vi "PJ_Edit_Freq.vi"() -> ()   [LabVIEW 2025]
uses:
  <vilib>/express/express analysis/Spectral/Block/exnSpectralBlock spectral measurements PSD poly.vi
  <vilib>/express/express analysis/Spectral/Block/exnSpectralBlock spectral measurements PSD DDT.vi
  <vilib>/express/express analysis/Spectral/XNode/ExpressSpectralMeasurementsBlockNode.xnode
panel:
  in  "start":bool
  in  "Boolean":bool
  in  "Fre":dbl
  in  "Am":dbl
  out "Clear4":bool
  out "Clear 3":bool
  out "Clear2":bool
  out "check":bool
  out "Clear1":bool
  out "com":bool
  out "call":bool
  out "ele":bool
  in  "Baseline":bool
  out "555":bool
  out "6 HZ 2":bool
  out "7 HZ":bool
  in  "Upper Cut-Off":dbl=40.0
  out "PSD":dynamicdata(graph)
  out "PSD MAX":dbl
  out "Index ที่มากที่สุด":i32
  out "max value":dbl
  out "B 22+1":dbl
  out "N 22+1":dbl
  in  "Aj 22+1":dbl
  out "B 22+1":dbl
  out "PSD 22+1":dbl
  out "B 22":dbl
  out "N 22":dbl
  in  "Aj 22":dbl
  out "B 22":dbl
  out "PSD 22":dbl
  out "B 22-1":dbl
  out "N 22-1":dbl
  in  "Aj 22-1":dbl
  out "B 22-1":dbl
  out "PSD 22-1":dbl
  out "9 Hz":dbl[](array[numeric])
  out "Max Index 9":i32
  out "PSD max 9":dbl
  out "PSD 11-1":dbl
  out "B 11-1":dbl
  in  "Aj 11-1":dbl
  out "N 11-1":dbl
  out "B 11-1":dbl
  out "PSD 11":dbl
  out "B 11":dbl
  in  "Aj 11":dbl
  out "N 11":dbl
  out "B 11":dbl
  out "PSD 11+1":dbl
  out "B 11+1":dbl
  in  "Aj 11+1":dbl
  out "N 11+1":dbl
  out "B 11+1":dbl
  out "8 Hz":dbl[](array[numeric])
  out "Max Index 8":i32
  out "PSD max 8":dbl
  out "B 16+1":dbl
  out "N 16+1":dbl
  in  "Aj  16+1":dbl
  out "B 16+1":dbl
  out "PSD  16+1":dbl
  out "B 16":dbl
  out "N  16":dbl
  in  "Aj  16":dbl
  out "B 16":dbl
  out "PSD  16":dbl
  out "B 16-1":dbl
  out "N  16-1":dbl
  in  "Aj   16-1":dbl
  out "B   16-1":dbl
  out "PSD 16-1":dbl
  out "B 8+1":dbl
  out "N 8+1":dbl
  in  "Aj  8+1":dbl
  out "B  8+1":dbl
  out "PSD 8+1":dbl
  out "B 8":dbl
  out "N  8":dbl
  in  "Aj  8":dbl
  out "B  8":dbl
  out "PSD 8":dbl
  out "B 8-1":dbl
  out "N  8-1":dbl
  in  "Aj  8-1":dbl
  out "B  8-1":dbl
  out "PSD 8-1":dbl
  out "PSD 14+1":dbl
  out "B 14+1":dbl
  in  "Aj 14+1":dbl
  out "N 14+1":dbl
  out "B 14+1":dbl
  out "PSD 14":dbl
  out "B 14":dbl
  in  "Aj 14":dbl
  out "N 14":dbl
  out "B 14":dbl
  out "PSD 14-1":dbl
  out "B 14-1":dbl
  in  "Aj 14-1":dbl
  out "N 14-1":dbl
  out "B 14-1":dbl
  out "PSD7+1":dbl
  out "B7+1":dbl
  in  "Aj7+1":dbl
  out "N7+1":dbl
  out "B7+1":dbl
  out "PSD 7":dbl
  out "B 7":dbl
  in  "Aj 7":dbl
  out "N7":dbl
  out "B7":dbl
  out "7 Hz":dbl[](array[numeric])
  out "Max Index 7":i32
  out "PSD max 7":dbl
  out "PSD 7-1":dbl
  out "B 7-1":dbl
  in  "Aj 7-1":dbl
  out "N7-1":dbl
  out "B7-1":dbl
  out "B12-1":dbl
  out "N12-1":dbl
  in  "Aj 12-1":dbl
  out "B 12-1":dbl
  out "PSD 12-1":dbl
  out "B12":dbl
  out "N12":dbl
  in  "Aj 12":dbl
  out "B12":dbl
  out "PSD 12":dbl
  out "B12+1":dbl
  out "N12+1":dbl
  in  "Aj 12+1":dbl
  out "B 12+1":dbl
  out "PSD 12+1":dbl
  out "B6+1":dbl
  out "N6+1":dbl
  in  "Aj 6+1":dbl
  out "B 6+1":dbl
  out "PSD 6+1":dbl
  out "B6":dbl
  out "N6":dbl
  in  "Aj 6":dbl
  out "B6":dbl
  out "PSD 6":dbl
  out "PSD 6-1":dbl
  out "6 Hz":dbl[](array[numeric])
  out "Max Index 6":i32
  out "PSD max 6":dbl
  out "B 6-1":dbl
  in  "Aj 6-1":dbl
  out "N6-1":dbl
  out "B6-1":dbl
  out "appended array":dbl[][](array[numeric])
  out "Filtered Signal":dynamicdata(graph)
  in  "Lower Cut-Off":dbl=1.0
  out "data":dynamicdata(graph) caption="Raw Data"
  in  "number of samples":i32=1000
  in  "rate":dbl=200.0 min=200.0 max=200.0
  out "?":bool
  out "?":bool
  out "?":bool
  out "?":bool
  out "?":bool
  out "?":bool
  out "?":bool
  out "?":bool
  out "?":bool
  out "?":bool
  out "?":bool=TRUE
  out "?":bool=TRUE
  out "?":bool=TRUE
  out "?":bool=TRUE
  out "?":bool=TRUE
  out "?":bool=TRUE
  out "?":bool=TRUE
  out "?":bool=TRUE
  out "?":bool=TRUE
  out "?":bool=TRUE
  out "?":bool
  out "?":bool
  out "?":bool
  out "?":bool
  out "?":bool
  out "?":bool
  out "?":bool
  out "?":bool
  out "?":bool
  out "?":bool
  out "?":bool=TRUE
  out "?":bool=TRUE
  out "?":bool=TRUE
  out "?":bool=TRUE
  out "?":bool=TRUE
  out "?":bool=TRUE
  out "?":bool=TRUE
  out "?":bool=TRUE
  out "?":bool=TRUE
  out "?":bool=TRUE
  out "?":bool
  out "?":bool
  out "?":bool
  out "?":bool
  out "?":bool
  out "?":bool
  out "?":bool
  out "?":bool
  out "?":bool
  out "?":bool
  out "?":bool=TRUE
  out "?":bool=TRUE
  out "?":bool=TRUE
  out "?":bool=TRUE
  out "?":bool=TRUE
  out "?":bool=TRUE
  out "?":bool=TRUE
  out "?":bool=TRUE
  out "?":bool=TRUE
  out "?":bool=TRUE
  out "?":bool
  out "?":bool
  out "?":bool
  out "?":bool
  out "?":bool
  out "?":bool
  out "?":bool
  out "?":bool
  out "?":bool
  out "?":bool
  out "?":bool=TRUE
  out "?":bool=TRUE
  out "?":bool=TRUE
  out "?":bool=TRUE
  out "?":bool=TRUE
  out "?":bool=TRUE
  out "?":bool=TRUE
  out "?":bool=TRUE
  out "?":bool=TRUE
  out "?":bool=TRUE
  out "9 HZ":bool
  out "8 HZ":bool
  in  "Tab Control":enum32{"TAB 1", "TAB 2", "TAB 3", "TAB 4"}(tab)
  out "Emotion 7":bool
  out "Emotion 6":bool
  out "Emotion 5":bool
  out "Emotion 4":bool
  out "ele":bool
  out "Emer":bool
  out "call":bool
  out "commu":bool
  out "Activity":bool
  out "8-2":bool
  out "commu_back":bool
  out "commu_2":bool
  out "commu_1":bool
  out "Emotion":bool
  out "ACC":bool
  out "back_page2":bool
  in  "send":bool
  out "call_back":bool
  out "call_3":bool
  out "call_back":bool
  out "call_2":bool
  out "call_1":bool
  out "1 3":bool
  out "1 2":bool
  out "1":bool
  out "String 2":string
  in  "SOS CALLING":bool
  in  "Search Button 2":bool
  out "ele_back":bool
  out "ele_3":bool
  out "ele_2":bool
  out "ele_1":bool
  out "ele_2":bool
  out "ele_3":bool
  out "ele_1":bool
  out "BACK_Page4":bool
  # "MENU"
  # "COMMUNICATION"
  # "SOS CALLING"
  # "Tel."
  # "ELECTRICAL DEVICES"
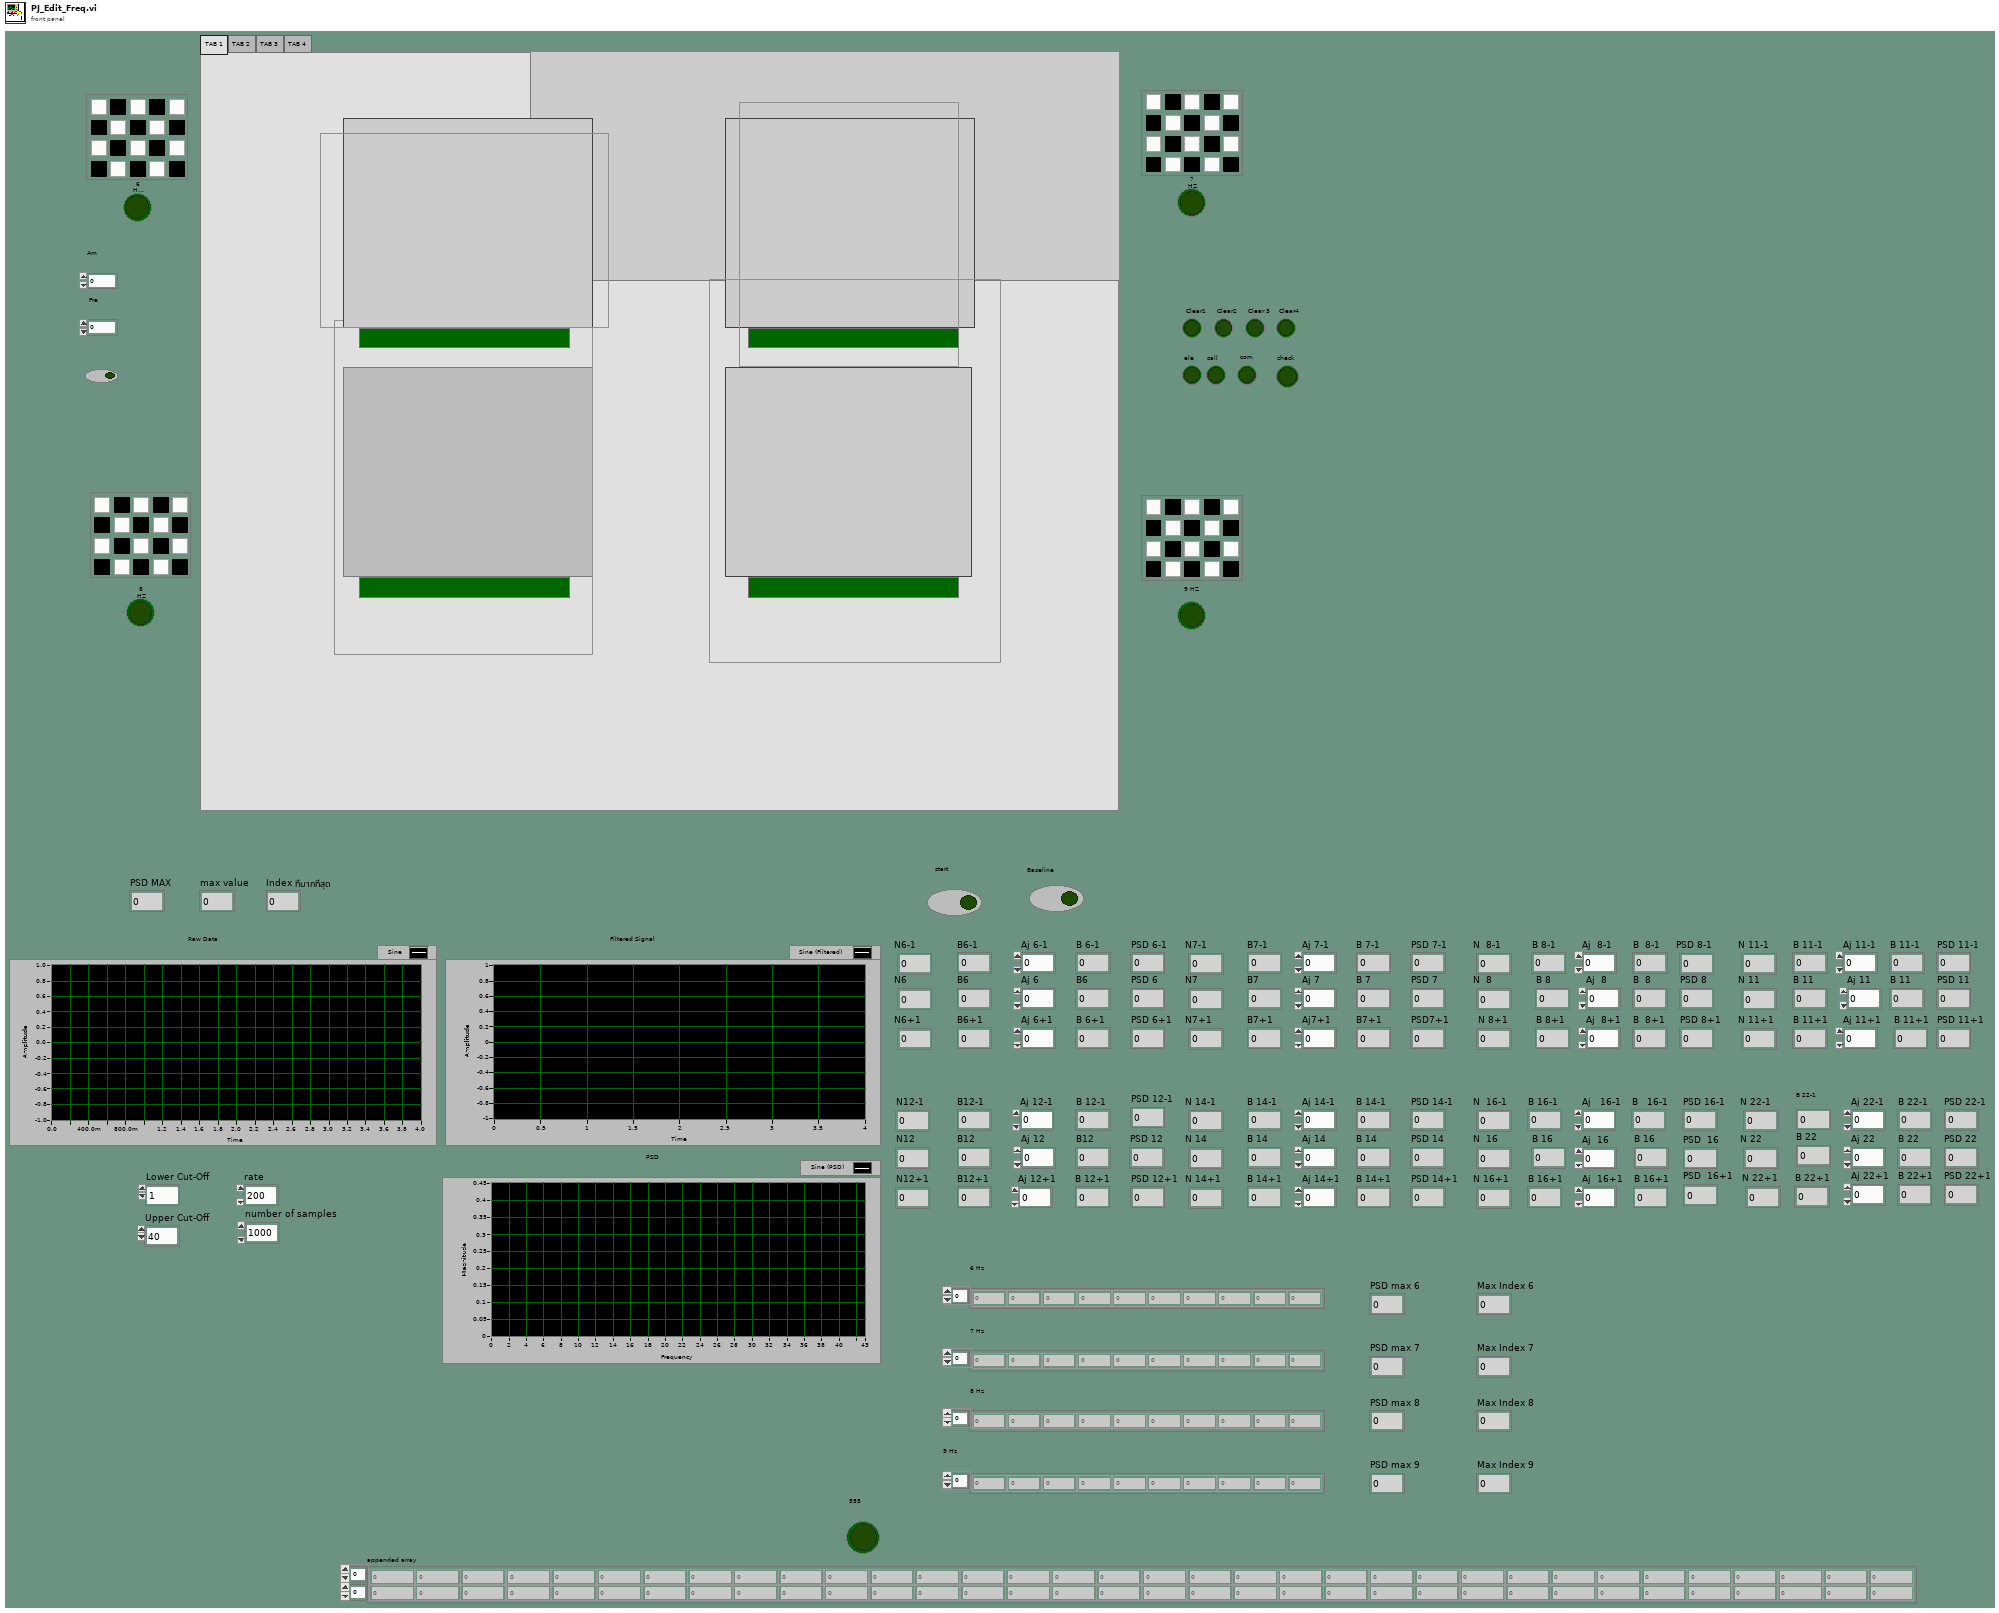
[diagram p1: front panel]
types:
  T1 = cluster{"averaging mode":u16, "weighting mode":u16, "number of averages":u32}
  T2 = cluster{"dB On (F)":bool, "unwrap phase (F)":bool, "convert to degree (F)":bool}
  T3 = enum32{"TAB 1", "TAB 2", "TAB 3", "TAB 4", "TAB 5", "TAB 6", "TAB 7"}
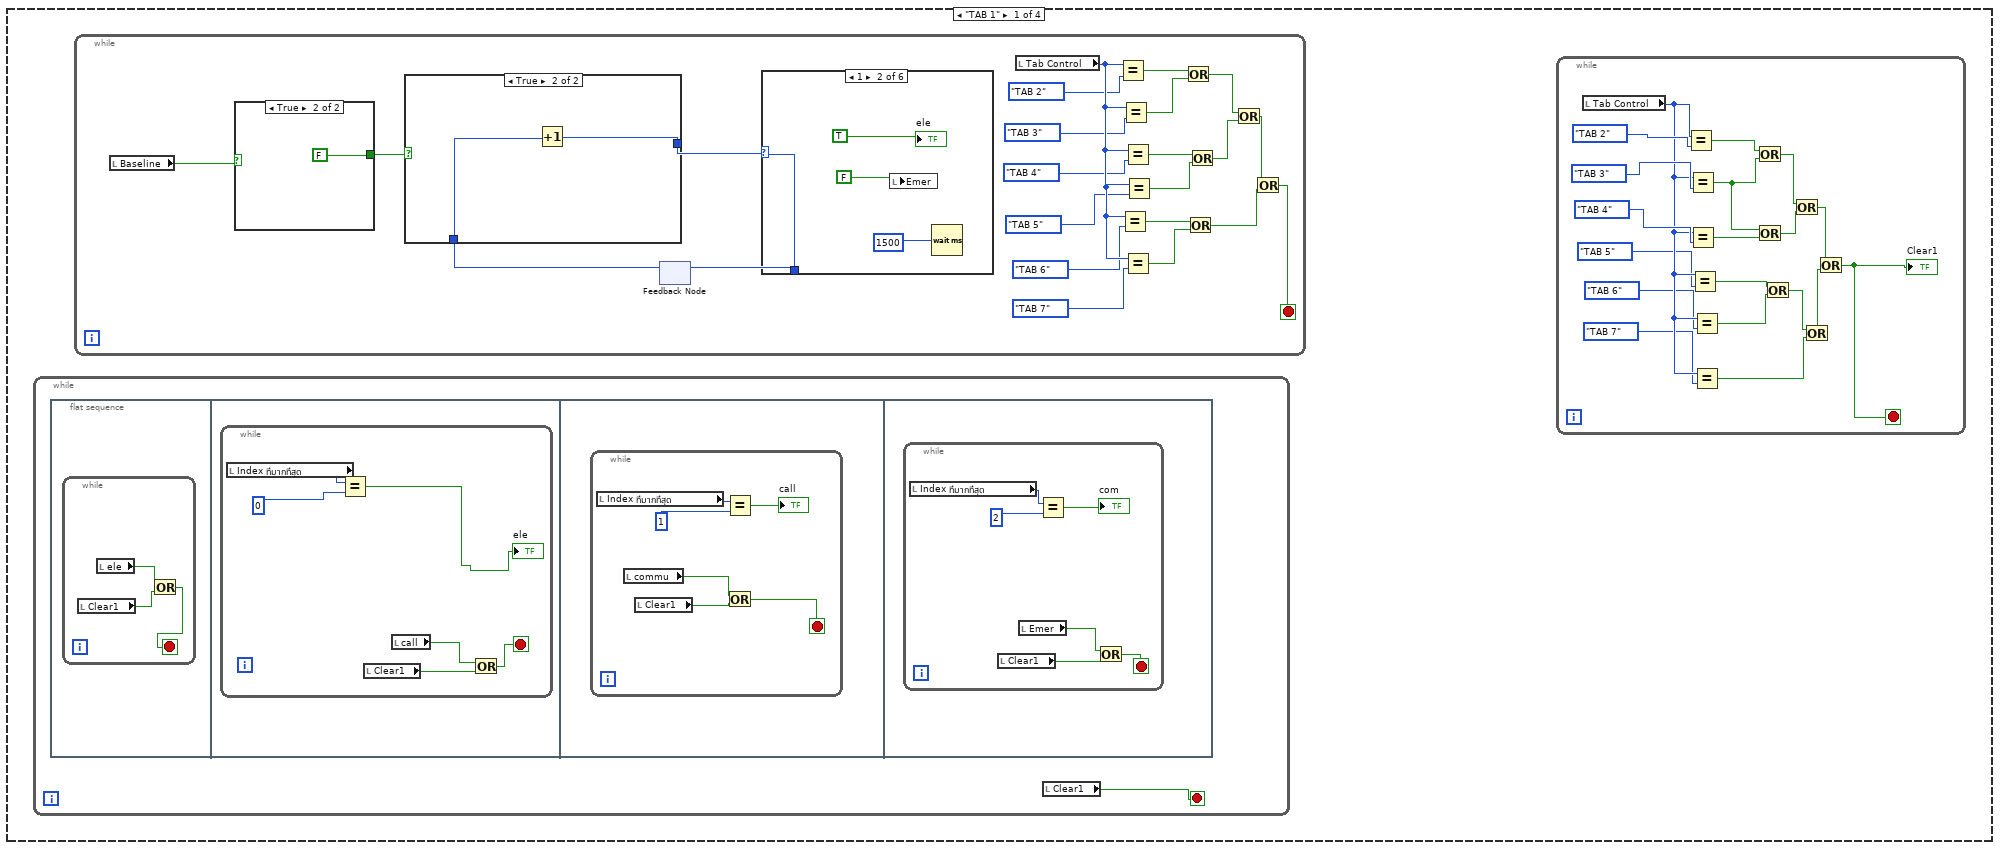
[diagram p2: hidden frame]
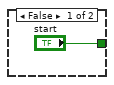
[diagram p3: hidden frame]
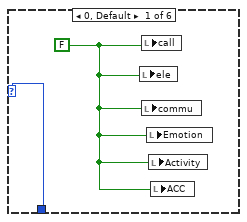
[diagram p4: hidden frame]
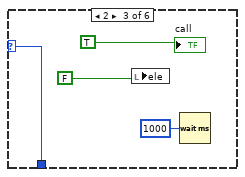
[diagram p5: hidden frame]
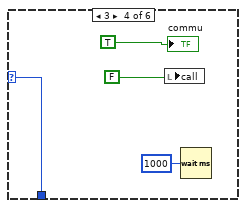
[diagram p6: hidden frame]
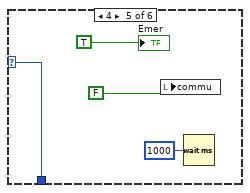
[diagram p7: hidden frame]
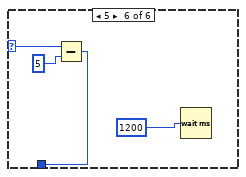
[diagram p8: hidden frame]
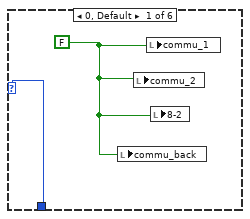
[diagram p10: hidden frame]
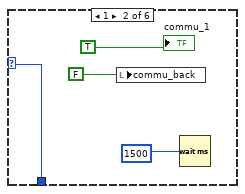
[diagram p11: hidden frame]
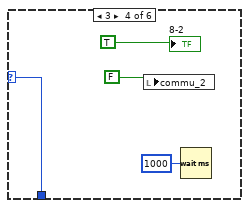
[diagram p12: hidden frame]
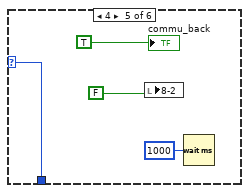
[diagram p13: hidden frame]
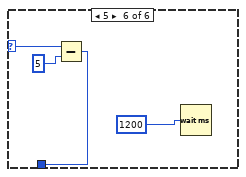
[diagram p14: hidden frame]
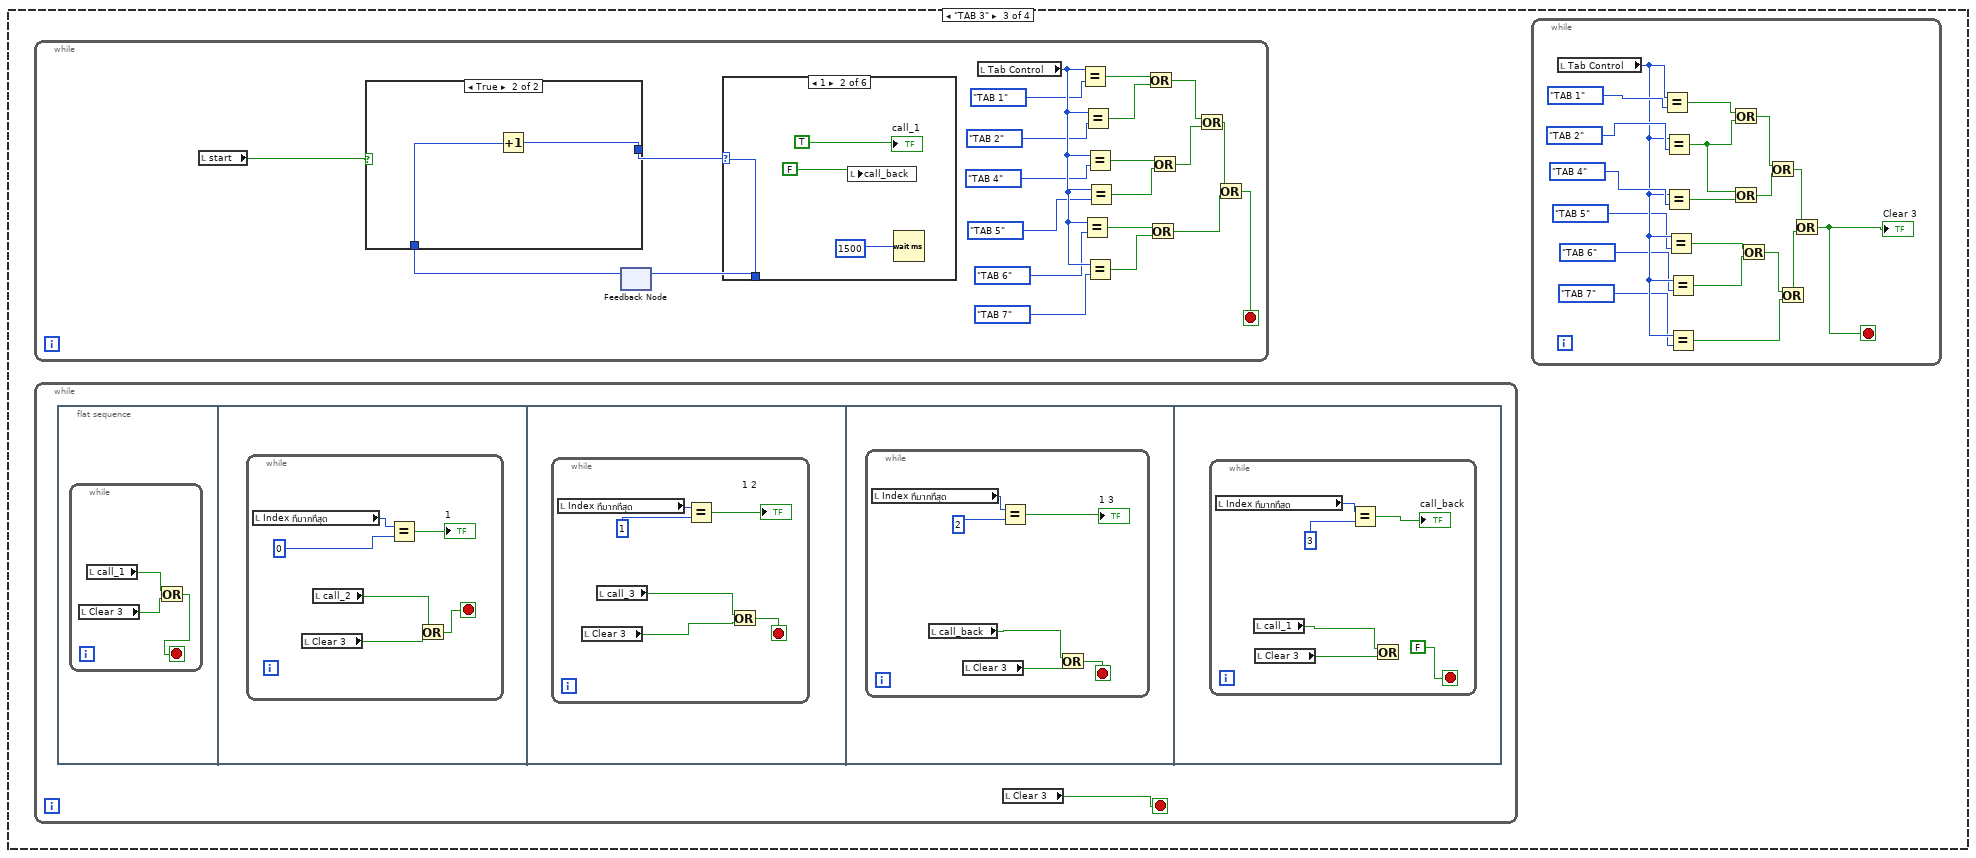
[diagram p16: hidden frame]
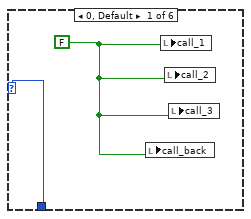
[diagram p17: hidden frame]
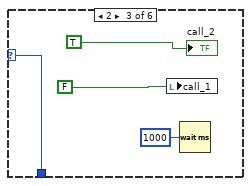
[diagram p18: hidden frame]
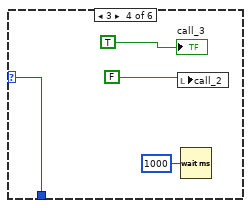
[diagram p19: hidden frame]
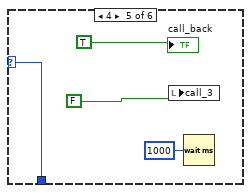
[diagram p20: hidden frame]
diagram:
  n1 = while {
    shift-right: [w7] -> _
    shift-left: "" -> [w9]
    stop <- FALSE stop-if-true
    n2 = event shown="[3] \"call_back\": Value Change" {
      selector: _ -> [_ _ _ _]
      dyn-events: _ -> [_ _ _ _]
      timeout: _ -> [_ _ _ _]
      tunnel: w9 -> [_ _ _ _]
      tunnel: ["0622436287" "1669" " 0937529340" _] -> w7
      event "1 2": Value Change {
        n3 = event-data() -> ()  [unwired: 1 in, 6 out]
      }
      event "1": Value Change {
        n4 = event-data() -> ()  [unwired: 1 in, 6 out]
      }
      event "1 3": Value Change {
        n5 = event-data() -> ()  [unwired: 1 in, 6 out]
      }
      event "call_back": Value Change {
        n6 = event-data() -> ()  [unwired: 1 in, 6 out]
        n7 = local write "Tab Control"(enum32{"TAB 1", "TAB 2", "TAB 3", "TAB 4"}."TAB 1" ("Tab Control")) -> ()
      }
    }
    "String 2" <- w7
  }
  n8 = while {
    stop <- FALSE stop-if-true
    n9 = while {
      stop <- FALSE stop-if-true
      n10 = while {
        stop <- FALSE stop-if-true
        w53 = 66.666667
        # "6 HZ"
        n11 = for {
          N: 2 -> [_]
          tunnel: w53 -> [w57]
          i -> [w59]
          n12 = Wait (ms)(milliseconds to wait=w57) -> ()  [unwired: 1 out]
          n13 = Equal?(x=0, y=w59) -> (x = y?=→"?" →"?" →"?" →"?" →"?" →"?" →"?" →"?" →"?" →"?":bool)
        }
        n14 = for {
          N: 2 -> [_]
          tunnel: w53 -> [w61]
          i -> [w62]
          n15 = Wait (ms)(milliseconds to wait=w61) -> ()  [unwired: 1 out]
          n16 = Equal?(x=1, y=w62) -> (x = y?=→"?" →"?" →"?" →"?" →"?" →"?" →"?" →"?" →"?" →"?":bool)
        }
      }
      n17 = while {
        stop <- FALSE stop-if-true
        w41 = 57.142857
        # "7 HZ"
        n18 = for {
          N: 2 -> [_]
          tunnel: w41 -> [w45]
          i -> [w47]
          n19 = Wait (ms)(milliseconds to wait=w45) -> ()  [unwired: 1 out]
          n20 = Equal?(x=0, y=w47) -> (x = y?=→"?" →"?" →"?" →"?" →"?" →"?" →"?" →"?" →"?" →"?":bool)
        }
        n21 = for {
          N: 2 -> [_]
          tunnel: w41 -> [w49]
          i -> [w50]
          n22 = Wait (ms)(milliseconds to wait=w49) -> ()  [unwired: 1 out]
          n23 = Equal?(x=1, y=w50) -> (x = y?=→"?" →"?" →"?" →"?" →"?" →"?" →"?" →"?" →"?" →"?":bool)
        }
      }
      n24 = while {
        stop <- FALSE stop-if-true
        w29 = 50.0
        # "8 HZ 50"
        n25 = for {
          N: 2 -> [_]
          tunnel: w29 -> [w33]
          i -> [w35]
          n26 = Wait (ms)(milliseconds to wait=w33) -> ()  [unwired: 1 out]
          n27 = Equal?(x=0, y=w35) -> (x = y?=→"?" →"?" →"?" →"?" →"?" →"?" →"?" →"?" →"?" →"?":bool)
        }
        n28 = for {
          N: 2 -> [_]
          tunnel: w29 -> [w37]
          i -> [w38]
          n29 = Wait (ms)(milliseconds to wait=w37) -> ()  [unwired: 1 out]
          n30 = Equal?(x=1, y=w38) -> (x = y?=→"?" →"?" →"?" →"?" →"?" →"?" →"?" →"?" →"?" →"?":bool)
        }
      }
      n31 = while {
        stop <- FALSE stop-if-true
        w17 = 36.3636363636
        # "11 36.36363636"
        # "9 HZ"
        n32 = for {
          N: 2 -> [_]
          tunnel: w17 -> [w21]
          i -> [w23]
          n33 = Wait (ms)(milliseconds to wait=w21) -> ()  [unwired: 1 out]
          n34 = Equal?(x=0, y=w23) -> (x = y?=→"?" →"?" →"?" →"?" →"?" →"?" →"?" →"?" →"?" →"?":bool)
        }
        n35 = for {
          N: 2 -> [_]
          tunnel: w17 -> [w25]
          i -> [w26]
          n36 = Wait (ms)(milliseconds to wait=w25) -> ()  [unwired: 1 out]
          n37 = Equal?(x=1, y=w26) -> (x = y?=→"?" →"?" →"?" →"?" →"?" →"?" →"?" →"?" →"?" →"?":bool)
        }
      }
    }
  }
  n38 = while {
    stop <- FALSE stop-if-true
    n39 = case shown="True" "Boolean" {
      tunnel: [w451 w457] -> w70
      tunnel: "Fre" -> [w452 w456]
      tunnel: "Am" -> [w453 w455]
      frame False {
        n40 = call "Simulate Signal2"("Frequency"=w452, "Amplitude"=w453) -> ("Sine"=w451:dynamicdata)  [unwired: 12 in, 1 out]
        n41 = Wait (ms)(milliseconds to wait=u32 1000) -> ()  [unwired: 1 out]
      }
      frame True {
        n42 = call "Simulate Signal"("Frequency"=w456, "Amplitude"=w455) -> ("Sine"=w457:dynamicdata)  [unwired: 12 in, 1 out]
        n43 = Wait (ms)(milliseconds to wait=u32 1000) -> ()  [unwired: 1 out]
      }
    }
    "data" <- w70
    n44 = Divide(x="number of samples", y="rate") -> (x/y=w160:dbl)
    n45 = call "Filter"("Lower Cut-Off"="Lower Cut-Off", "Upper Cut-Off"="Upper Cut-Off", "Signal"=w70) -> ("Filtered Signal"=w75:dynamicdata)  [unwired: 7 in, 1 out]
    "Filtered Signal" <- w75
    n46 = Divide(x=8.0, y=w160) -> (x/y=w260:dbl)
    n47 = Divide(x=16.0, y=w160) -> (x/y=w212:dbl)
    n48 = Divide(x=14.0, y=w160) -> (x/y=w285:dbl)
    n49 = Divide(x=22.0, y=w160) -> (x/y=w135:dbl)
    n50 = xnode "Spectral Measurements"("Signals"=w75) -> ("PSD"=w101:dynamicdata)  [unwired: 1 in, 1 out]
    "PSD" <- w101
    n51 = Divide(x=11.0, y=w160) -> (x/y=w178:dbl)
    n52 = Divide(x=7.0, y=w160) -> (x/y=w302:dbl)
    n53 = Divide(x=12.0, y=w160) -> (x/y=w371:dbl)
    n54 = Divide(x=6.0, y=w160) -> (x/y=w420:dbl)
    n55 = call "Convert from Dynamic Data"("Dynamic Data Type"=w101) -> ("Array"=w448:dbl[])  [unwired: 3 in]
    n56 = Decrement(x=w178) -> (x-1=w209:dbl)
    n57 = Increment(x=w178) -> (x+1=w177:dbl)
    n58 = Increment(x=w135) -> (x+1=w124:dbl)
    n59 = Decrement(x=w135) -> (x-1=w149:dbl)
    n60 = Decrement(x=w285) -> (x-1=w314:dbl)
    n61 = Increment(x=w260) -> (x+1=w250:dbl)
    n62 = Decrement(x=w212) -> (x-1=w235:dbl)
    n63 = Decrement(x=w420) -> (x-1=w433:dbl)
    n64 = Decrement(x=w302) -> (x-1=w343:dbl)
    "PSD 7-1" <- w343
    n65 = Increment(x=w302) -> (x+1=w328:dbl)
    n66 = Decrement(x=w260) -> (x-1=w273:dbl)
    n67 = Increment(x=w212) -> (x+1=w211:dbl)
    n68 = Increment(x=w420) -> (x+1=w409:dbl)
    n69 = Increment(x=w285) -> (x+1=w291:dbl)
    n70 = Decrement(x=w371) -> (x-1=w376:dbl)
    n71 = Increment(x=w371) -> (x+1=w370:dbl)
    n72 = Build Array(w448) -> (w125:dbl[][])
    "appended array" <- w125
    n73 = Index Array(array=w125, index (row)=0, index (col)=w235) -> (element=w246:dbl)
    "PSD 16-1" <- w246
    n74 = Index Array(array=w125, index (row)=0 ("disabled index (row)"), index (col)=w211) -> (element=w223:dbl)
    "PSD  16+1" <- w223
    n75 = Index Array(array=w125, index (row)=0 ("disabled index (row)"), index (col)=w212) -> (element=w225:dbl)
    "PSD  16" <- w225
    n76 = Index Array(array=w125, index (row)=0, index (col)=w291) -> (element=w292:dbl)
    "PSD 14+1" <- w292
    n77 = Index Array(array=w125, index (row)=0 ("disabled index (row)"), index (col)=w149) -> (element=w147:dbl)
    "PSD 22-1" <- w147
    n78 = Index Array(array=w125, index (row)=0, index (col)=w250) -> (element=w248:dbl)
    "PSD 8+1" <- w248
    n79 = Index Array(array=w125, index (row)=0 ("disabled index (row)"), index (col)=w124) -> (element=w122:dbl)
    "PSD 22+1" <- w122
    n80 = Index Array(array=w125, index (row)=0, index (col)=w177) -> (element=w166:dbl)
    "PSD 11-1" <- w166
    n81 = Index Array(array=w125, index (row)=0, index (col)=w260) -> (element=w271:dbl)
    "PSD 8" <- w271
    n82 = Index Array(array=w125, index (row)=0 ("disabled index (row)"), index (col)=w135) -> (element=w136:dbl)
    "PSD 22" <- w136
    n83 = Index Array(array=w125, index (row)=0, index (col)=w273) -> (element=w272:dbl)
    "PSD 8-1" <- w272
    n84 = Index Array(array=w125, index (row)=0, index (col)=w178) -> (element=w179:dbl)
    "PSD 11" <- w179
    n85 = Index Array(array=w125, index (row)=0, index (col)=w209) -> (element=w190:dbl)
    "PSD 11+1" <- w190
    n86 = Index Array(array=w125, index (row)=0, index (col)=w314) -> (element=w316:dbl)
    "PSD 14-1" <- w316
    n87 = Index Array(array=w125, index (row)=0, index (col)=w285) -> (element=w303:dbl)
    "PSD 14" <- w303
    n88 = Index Array(array=w125, index (row)=0, index (col)=w343) -> ()  [unwired: 1 out]
    n89 = Index Array(array=w125, index (row)=0 ("disabled index (row)"), index (col)=w302) -> (element=w340:dbl)
    "PSD 7" <- w340
    n90 = Index Array(array=w125, index (row)=0, index (col)=w328) -> (element=w329:dbl)
    "PSD7+1" <- w329
    n91 = Index Array(array=w125, index (row)=0 ("disabled index (row)"), index (col)=w409) -> (element=w407:dbl)
    "PSD 6+1" <- w407
    n92 = Index Array(array=w125, index (row)=0, index (col)=w376) -> (element=w375:dbl)
    "PSD 12-1" <- w375
    n93 = Index Array(array=w125, index (row)=0 ("disabled index (row)"), index (col)=w371) -> (element=w372:dbl)
    "PSD 12" <- w372
    n94 = Index Array(array=w125, index (row)=0 ("disabled index (row)"), index (col)=w370) -> (element=w368:dbl)
    "PSD 12+1" <- w368
    n95 = Index Array(array=w125, index (row)=0, index (col)=w420) -> (element=w421:dbl)
    "PSD 6" <- w421
    n96 = Index Array(array=w125, index (row)=0, index (col)=w433) -> (element=w440:dbl)
    "PSD 6-1" <- w440
    n97 = feedback #1() -> (w77:dbl)  [unwired: 1 in]
    "B 22" <- w77
    n98 = case shown="False" "Baseline" {
      tunnel: w136 -> [_ w467]
      tunnel: [w466 w467] -> w138
      tunnel: w77 -> [w466 _]
      frame False {
      }
      frame True {
      }
    }
    n99 = feedback-in #1(w138) -> ()
    n100 = feedback #2() -> (w78:dbl)  [unwired: 1 in]
    "B 22-1" <- w78
    n101 = case shown="False" "Baseline" {
      tunnel: w147 -> [_ w471]
      tunnel: [w470 w471] -> w158
      tunnel: w78 -> [w470 _]
      frame False {
      }
      frame True {
      }
    }
    n102 = feedback-in #2(w158) -> ()
    n103 = feedback #3() -> (w76:dbl)  [unwired: 1 in]
    "B 22+1" <- w76
    n104 = case shown="False" "Baseline" {
      tunnel: w122 -> [_ w463]
      tunnel: [w462 w463] -> w134
      tunnel: w76 -> [w462 _]
      frame False {
      }
      frame True {
      }
    }
    n105 = feedback-in #3(w134) -> ()
    n106 = feedback #4() -> (w84:dbl)  [unwired: 1 in]
    "B 16-1" <- w84
    n107 = case shown="True" "Baseline" {
      tunnel: w246 -> [_ w495]
      tunnel: [w494 w495] -> w236
      tunnel: w84 -> [w494 _]
      frame False {
      }
      frame True {
      }
    }
    n108 = feedback-in #4(w236) -> ()
    n109 = feedback #5() -> (w82:dbl)  [unwired: 1 in]
    "B 16+1" <- w82
    n110 = case shown="True" "Baseline" {
      tunnel: w223 -> [_ w487]
      tunnel: [w486 w487] -> w214
      tunnel: w82 -> [w486 _]
      frame False {
      }
      frame True {
      }
    }
    n111 = feedback-in #5(w214) -> ()
    n112 = feedback #6() -> (w83:dbl)  [unwired: 1 in]
    "B 16" <- w83
    n113 = case shown="True" "Baseline" {
      tunnel: w225 -> [_ w491]
      tunnel: [w490 w491] -> w234
      tunnel: w83 -> [w490 _]
      frame False {
      }
      frame True {
      }
    }
    n114 = feedback-in #6(w234) -> ()
    n115 = feedback #7() -> (w85:dbl)  [unwired: 1 in]
    "B 8+1" <- w85
    n116 = case shown="True" "Baseline" {
      tunnel: w248 -> [_ w499]
      tunnel: [w498 w499] -> w259
      tunnel: w85 -> [w498 _]
      frame False {
      }
      frame True {
      }
    }
    n117 = feedback-in #7(w259) -> ()
    n118 = feedback #8() -> (w88:dbl)  [unwired: 1 in]
    "B 14+1" <- w88
    n119 = case shown="True" "Baseline" {
      tunnel: w292 -> [_ w511]
      tunnel: [w510 w511] -> w293
      tunnel: w88 -> [w510 _]
      frame False {
      }
      frame True {
      }
    }
    n120 = feedback-in #8(w293) -> ()
    n121 = feedback #9() -> (w86:dbl)  [unwired: 1 in]
    "B 8" <- w86
    n122 = case shown="True" "Baseline" {
      tunnel: w271 -> [_ w503]
      tunnel: [w502 w503] -> w262
      tunnel: w86 -> [w502 _]
      frame False {
      }
      frame True {
      }
    }
    n123 = feedback-in #9(w262) -> ()
    n124 = feedback #10() -> (w80:dbl)  [unwired: 1 in]
    "B 11" <- w80
    n125 = case shown="False" "Baseline" {
      tunnel: w179 -> [_ w479]
      tunnel: [w478 w479] -> w180
      tunnel: w80 -> [w478 _]
      frame False {
      }
      frame True {
      }
    }
    n126 = feedback-in #10(w180) -> ()
    n127 = feedback #11() -> (w87:dbl)  [unwired: 1 in]
    "B 8-1" <- w87
    n128 = case shown="True" "Baseline" {
      tunnel: w272 -> [_ w507]
      tunnel: [w506 w507] -> w283
      tunnel: w87 -> [w506 _]
      frame False {
      }
      frame True {
      }
    }
    n129 = feedback-in #11(w283) -> ()
    n130 = feedback #12() -> (w81:dbl)  [unwired: 1 in]
    "B 11+1" <- w81
    n131 = case shown="True" "Baseline" {
      tunnel: w190 -> [_ w483]
      tunnel: [w482 w483] -> w191
      tunnel: w81 -> [w482 _]
      frame False {
      }
      frame True {
      }
    }
    n132 = feedback-in #12(w191) -> ()
    n133 = feedback #13() -> (w96:dbl)  [unwired: 1 in]
    "B12-1" <- w96
    n134 = case shown="True" "Baseline" {
      tunnel: w375 -> [_ w543]
      tunnel: [w542 w543] -> w387
      tunnel: w96 -> [w542 _]
      frame False {
      }
      frame True {
      }
    }
    n135 = feedback-in #13(w387) -> ()
    n136 = feedback #14() -> (w90:dbl)  [unwired: 1 in]
    "B 14-1" <- w90
    n137 = case shown="True" "Baseline" {
      tunnel: w316 -> [_ w519]
      tunnel: [w518 w519] -> w317
      tunnel: w90 -> [w518 _]
      frame False {
      }
      frame True {
      }
    }
    n138 = feedback-in #14(w317) -> ()
    n139 = feedback #15() -> (w79:dbl)  [unwired: 1 in]
    "B 11-1" <- w79
    n140 = case shown="False" "Baseline" {
      tunnel: w166 -> [_ w475]
      tunnel: [w474 w475] -> w167
      tunnel: w79 -> [w474 _]
      frame False {
      }
      frame True {
      }
    }
    n141 = feedback-in #15(w167) -> ()
    n142 = feedback #16() -> (w97:dbl)  [unwired: 1 in]
    "B6+1" <- w97
    n143 = case shown="True" "Baseline" {
      tunnel: w407 -> [_ w547]
      tunnel: [w546 w547] -> w410
      tunnel: w97 -> [w546 _]
      frame False {
      }
      frame True {
      }
    }
    n144 = feedback-in #16(w410) -> ()
    n145 = feedback #17() -> (w98:dbl)  [unwired: 1 in]
    "B6" <- w98
    n146 = case shown="True" "Baseline" {
      tunnel: w421 -> [_ w551]
      tunnel: [w550 w551] -> w431
      tunnel: w98 -> [w550 _]
      frame False {
      }
      frame True {
      }
    }
    n147 = feedback-in #17(w431) -> ()
    n148 = feedback #18() -> (w99:dbl)  [unwired: 1 in]
    "B6-1" <- w99
    n149 = case shown="False" "Baseline" {
      tunnel: w440 -> [_ w555]
      tunnel: [w554 w555] -> w432
      tunnel: w99 -> [w554 _]
      frame False {
      }
      frame True {
      }
    }
    n150 = feedback-in #18(w432) -> ()
    n151 = feedback #19() -> (w89:dbl)  [unwired: 1 in]
    "B 14" <- w89
    n152 = case shown="True" "Baseline" {
      tunnel: w303 -> [_ w515]
      tunnel: [w514 w515] -> w305
      tunnel: w89 -> [w514 _]
      frame False {
      }
      frame True {
      }
    }
    n153 = feedback-in #19(w305) -> ()
    n154 = feedback #20() -> (w94:dbl)  [unwired: 1 in]
    "B12+1" <- w94
    n155 = case shown="True" "Baseline" {
      tunnel: w368 -> [_ w535]
      tunnel: [w534 w535] -> w405
      tunnel: w94 -> [w534 _]
      frame False {
      }
      frame True {
      }
    }
    n156 = feedback-in #20(w405) -> ()
    n157 = Add(x=w77, y="Aj 22") -> (x+y=w142:dbl)
    "B 22" <- w142
    n158 = Add(x=w78, y="Aj 22-1") -> (x+y=w154:dbl)
    "B 22-1" <- w154
    n159 = Add(x=w76, y="Aj 22+1") -> (x+y=w130:dbl)
    "B 22+1" <- w130
    n160 = feedback #21() -> (w95:dbl)  [unwired: 1 in]
    "B12" <- w95
    n161 = case shown="True" "Baseline" {
      tunnel: w372 -> [_ w539]
      tunnel: [w538 w539] -> w388
      tunnel: w95 -> [w538 _]
      frame False {
      }
      frame True {
      }
    }
    n162 = feedback-in #21(w388) -> ()
    n163 = Add(x=w84, y="Aj   16-1") -> (x+y=w240:dbl)
    "B   16-1" <- w240
    n164 = Add(x=w82, y="Aj  16+1") -> (x+y=w218:dbl)
    "B 16+1" <- w218
    n165 = Add(x=w83, y="Aj  16") -> (x+y=w230:dbl)
    "B 16" <- w230
    n166 = Add(x=w85, y="Aj  8+1") -> (x+y=w255:dbl)
    "B  8+1" <- w255
    n167 = Add(x=w88, y="Aj 14+1") -> (x+y=w297:dbl)
    "B 14+1" <- w297
    n168 = Add(x=w86, y="Aj  8") -> (x+y=w266:dbl)
    "B  8" <- w266
    n169 = Add(x=w80, y="Aj 11") -> (x+y=w184:dbl)
    "B 11" <- w184
    n170 = Add(x=w87, y="Aj  8-1") -> (x+y=w279:dbl)
    "B  8-1" <- w279
    n171 = Add(x=w81, y="Aj 11+1") -> (x+y=w195:dbl)
    "B 11+1" <- w195
    n172 = Add(x=w96, y="Aj 12-1") -> (x+y=w383:dbl)
    "B 12-1" <- w383
    n173 = Add(x=w90, y="Aj 14-1") -> (x+y=w321:dbl)
    "B 14-1" <- w321
    n174 = Add(x=w79, y="Aj 11-1") -> (x+y=w171:dbl)
    "B 11-1" <- w171
    n175 = Multiply(x=w77, y=4.0) -> (x*y=w145:dbl)
    "N 22" <- w145
    n176 = Add(x=w97, y="Aj 6+1") -> (x+y=w414:dbl)
    "B 6+1" <- w414
    n177 = Multiply(x=w78, y=4.0) -> (x*y=w151:dbl)
    "N 22-1" <- w151
    n178 = Multiply(x=w76, y=4.0) -> (x*y=w127:dbl)
    "N 22+1" <- w127
    n179 = feedback #22() -> (w91:dbl)  [unwired: 1 in]
    "B7+1" <- w91
    n180 = case shown="True" "Baseline" {
      tunnel: w329 -> [_ w523]
      tunnel: [w522 w523] -> w331
      tunnel: w91 -> [w522 _]
      frame False {
      }
      frame True {
      }
    }
    n181 = feedback-in #22(w331) -> ()
    n182 = feedback #23() -> (w92:dbl)  [unwired: 1 in]
    "B7" <- w92
    n183 = case shown="True" "Baseline" {
      tunnel: w340 -> [_ w527]
      tunnel: [w526 w527] -> w344
      tunnel: w92 -> [w526 _]
      frame False {
      }
      frame True {
      }
    }
    n184 = feedback-in #23(w344) -> ()
    n185 = Multiply(x=w84, y=4.0) -> (x*y=w243:dbl)
    "N  16-1" <- w243
    n186 = Multiply(x=w82, y=4.0) -> (x*y=w221:dbl)
    "N 16+1" <- w221
    n187 = Multiply(x=w83, y=4.0) -> (x*y=w227:dbl)
    "N  16" <- w227
    n188 = Multiply(x=w85, y=4.0) -> (x*y=w252:dbl)
    "N 8+1" <- w252
    n189 = feedback #24() -> (w93:dbl)  [unwired: 1 in]
    "B7-1" <- w93
    n190 = case shown="True" "Baseline" {
      tunnel: w343 -> [_ w531]
      tunnel: [w530 w531] -> w357
      tunnel: w93 -> [w530 _]
      frame False {
      }
      frame True {
      }
    }
    n191 = feedback-in #24(w357) -> ()
    n192 = Add(x=w98, y="Aj 6") -> (x+y=w427:dbl)
    "B6" <- w427
    n193 = Add(x=w99, y="Aj 6-1") -> (x+y=w441:dbl)
    "B 6-1" <- w441
    n194 = Add(x=w89, y="Aj 14") -> (x+y=w309:dbl)
    "B 14" <- w309
    n195 = Multiply(x=w88, y=4.0) -> (x*y=w300:dbl)
    "N 14+1" <- w300
    n196 = Multiply(x=w86, y=4.0) -> (x*y=w269:dbl)
    "N  8" <- w269
    n197 = Multiply(x=w80, y=4.0) -> (x*y=w187:dbl)
    "N 11" <- w187
    n198 = Multiply(x=w87, y=4.0) -> (x*y=w276:dbl)
    "N  8-1" <- w276
    n199 = Multiply(x=w81, y=4.0) -> (x*y=w198:dbl)
    "N 11+1" <- w198
    n200 = Add(x=w94, y="Aj 12+1") -> (x+y=w401:dbl)
    "B 12+1" <- w401
    n201 = Multiply(x=w96, y=4.0) -> (x*y=w380:dbl)
    "N12-1" <- w380
    n202 = Multiply(x=w90, y=4.0) -> (x*y=w324:dbl)
    "N 14-1" <- w324
    n203 = Add(x=w95, y="Aj 12") -> (x+y=w392:dbl)
    "B12" <- w392
    n204 = Multiply(x=w79, y=4.0) -> (x*y=w174:dbl)
    "N 11-1" <- w174
    n205 = Multiply(x=w97, y=4.0) -> (x*y=w417:dbl)
    "N6+1" <- w417
    n206 = Greater?(x=w136, y=w142) -> (0:w143:bool)
    n207 = Greater?(x=w147, y=w154) -> (0:w153:bool)
    n208 = Greater?(x=w122, y=w130) -> (0:w129:bool)
    n209 = Less?(x=w136, y=w145) -> (x < y?=w144:bool)
    n210 = Less?(x=w147, y=w151) -> (x < y?=w152:bool)
    n211 = Multiply(x=w98, y=4.0) -> (x*y=w424:dbl)
    "N6" <- w424
    n212 = Multiply(x=w99, y=4.0) -> (x*y=w444:dbl)
    "N6-1" <- w444
    n213 = Multiply(x=w89, y=4.0) -> (x*y=w312:dbl)
    "N 14" <- w312
    n214 = Greater?(x=w246, y=w240) -> (0:w241:bool)
    n215 = Less?(x=w122, y=w127) -> (x < y?=w128:bool)
    n216 = Greater?(x=w223, y=w218) -> (0:w219:bool)
    n217 = Greater?(x=w225, y=w230) -> (0:w229:bool)
    n218 = Greater?(x=w248, y=w255) -> (0:w254:bool)
    n219 = Less?(x=w246, y=w243) -> (x < y?=w242:bool)
    n220 = Less?(x=w223, y=w221) -> (x < y?=w220:bool)
    n221 = Multiply(x=w94, y=4.0) -> (x*y=w398:dbl)
    "N12+1" <- w398
    n222 = Less?(x=w225, y=w227) -> (x < y?=w228:bool)
    n223 = Greater?(x=w292, y=w297) -> (0:w298:bool)
    n224 = Less?(x=w248, y=w252) -> (x < y?=w253:bool)
    n225 = Greater?(x=w271, y=w266) -> (0:w267:bool)
    n226 = Greater?(x=w179, y=w184) -> (0:w185:bool)
    n227 = Multiply(x=w95, y=4.0) -> (x*y=w395:dbl)
    "N12" <- w395
    n228 = Add(x=w91, y="Aj7+1") -> (x+y=w335:dbl)
    "B7+1" <- w335
    n229 = Less?(x=w292, y=w300) -> (x < y?=w299:bool)
    n230 = Greater?(x=w272, y=w279) -> (0:w278:bool)
    n231 = Less?(x=w271, y=w269) -> (x < y?=w268:bool)
    n232 = Less?(x=w179, y=w187) -> (x < y?=w186:bool)
    n233 = Greater?(x=w190, y=w195) -> (0:w196:bool)
    n234 = Add(x=w92, y="Aj 7") -> (x+y=w348:dbl)
    "B 7" <- w348
    n235 = Less?(x=w272, y=w276) -> (x < y?=w277:bool)
    n236 = Greater?(x=w375, y=w383) -> (0:w382:bool)
    n237 = Greater?(x=w316, y=w321) -> (0:w322:bool)
    n238 = Less?(x=w190, y=w198) -> (x < y?=w197:bool)
    n239 = Greater?(x=w166, y=w171) -> (0:w172:bool)
    n240 = Add(x=w93, y="Aj 7-1") -> (x+y=w361:dbl)
    "B 7-1" <- w361
    n241 = Greater?(x=w407, y=w414) -> (0:w415:bool)
    n242 = Less?(x=w375, y=w380) -> (x < y?=w381:bool)
    n243 = Less?(x=w316, y=w324) -> (x < y?=w323:bool)
    n244 = Less?(x=w166, y=w174) -> (x < y?=w173:bool)
    n245 = Less?(x=w407, y=w417) -> (x < y?=w416:bool)
    n246 = And(x=w144, y=w143) -> (x .and. y?=w141:bool)
    n247 = Subtract(x=w136, y=w142) -> (x-y=w140:dbl)
    n248 = And(x=w152, y=w153) -> (x .and. y?=w155:bool)
    n249 = Greater?(x=w421, y=w427) -> (0:w426:bool)
    n250 = Subtract(x=w147, y=w154) -> (x-y=w156:dbl)
    n251 = Greater?(x=w440, y=w441) -> (0:w442:bool)
    n252 = Greater?(x=w303, y=w309) -> (0:w310:bool)
    n253 = And(x=w128, y=w129) -> (x .and. y?=w131:bool)
    n254 = Subtract(x=w122, y=w130) -> (x-y=w132:dbl)
    n255 = Less?(x=w421, y=w424) -> (x < y?=w425:bool)
    n256 = Less?(x=w440, y=w444) -> (x < y?=w443:bool)
    n257 = Less?(x=w303, y=w312) -> (x < y?=w311:bool)
    n258 = And(x=w242, y=w241) -> (x .and. y?=w239:bool)
    n259 = Multiply(x=w91, y=4.0) -> (x*y=w338:dbl)
    "N7+1" <- w338
    n260 = Subtract(x=w246, y=w240) -> (x-y=w238:dbl)
    n261 = And(x=w220, y=w219) -> (x .and. y?=w217:bool)
    n262 = Subtract(x=w223, y=w218) -> (x-y=w216:dbl)
    n263 = Greater?(x=w368, y=w401) -> (0:w400:bool)
    n264 = Multiply(x=w92, y=4.0) -> (x*y=w351:dbl)
    "N7" <- w351
    n265 = And(x=w228, y=w229) -> (x .and. y?=w231:bool)
    n266 = And(x=w253, y=w254) -> (x .and. y?=w256:bool)
    n267 = Subtract(x=w225, y=w230) -> (x-y=w232:dbl)
    n268 = Subtract(x=w248, y=w255) -> (x-y=w257:dbl)
    n269 = Greater?(x=w372, y=w392) -> (0:w393:bool)
    n270 = Less?(x=w368, y=w398) -> (x < y?=w399:bool)
    n271 = And(x=w299, y=w298) -> (x .and. y?=w296:bool)
    n272 = Subtract(x=w292, y=w297) -> (x-y=w295:dbl)
    n273 = Multiply(x=w93, y=4.0) -> (x*y=w364:dbl)
    "N7-1" <- w364
    n274 = And(x=w268, y=w267) -> (x .and. y?=w265:bool)
    n275 = Subtract(x=w271, y=w266) -> (x-y=w264:dbl)
    n276 = And(x=w186, y=w185) -> (x .and. y?=w183:bool)
    n277 = Subtract(x=w179, y=w184) -> (x-y=w182:dbl)
    n278 = Less?(x=w372, y=w395) -> (x < y?=w394:bool)
    n279 = And(x=w277, y=w278) -> (x .and. y?=w280:bool)
    n280 = Subtract(x=w272, y=w279) -> (x-y=w281:dbl)
    n281 = And(x=w197, y=w196) -> (x .and. y?=w194:bool)
    n282 = Subtract(x=w190, y=w195) -> (x-y=w193:dbl)
    n283 = And(x=w381, y=w382) -> (x .and. y?=w384:bool)
    n284 = Subtract(x=w375, y=w383) -> (x-y=w385:dbl)
    n285 = And(x=w323, y=w322) -> (x .and. y?=w320:bool)
    n286 = Subtract(x=w316, y=w321) -> (x-y=w319:dbl)
    n287 = And(x=w173, y=w172) -> (x .and. y?=w170:bool)
    n288 = Subtract(x=w166, y=w171) -> (x-y=w169:dbl)
    n289 = Subtract(x=w407, y=w414) -> (x-y=w412:dbl)
    n290 = And(x=w416, y=w415) -> (x .and. y?=w413:bool)
    n291 = And(x=w443, y=w442) -> (x .and. y?=w439:bool)
    n292 = Subtract(x=w421, y=w427) -> (x-y=w429:dbl)
    n293 = And(x=w311, y=w310) -> (x .and. y?=w308:bool)
    n294 = Subtract(x=w440, y=w441) -> (x-y=w438:dbl)
    n295 = Greater?(x=w329, y=w335) -> (0:w336:bool)
    n296 = Subtract(x=w303, y=w309) -> (x-y=w307:dbl)
    n297 = Greater?(x=w340, y=w348) -> (0:w349:bool)
    n298 = And(x=w425, y=w426) -> (x .and. y?=w428:bool)
    n299 = Less?(x=w329, y=w338) -> (x < y?=w337:bool)
    n300 = Less?(x=w340, y=w351) -> (x < y?=w350:bool)
    n301 = Subtract(x=w368, y=w401) -> (x-y=w403:dbl)
    n302 = Greater?(x=w343, y=w361) -> (0:w362:bool)
    n303 = Subtract(x=w372, y=w392) -> (x-y=w390:dbl)
    n304 = And(x=w399, y=w400) -> (x .and. y?=w402:bool)
    n305 = Less?(x=w343, y=w364) -> (x < y?=w363:bool)
    n306 = And(x=w394, y=w393) -> (x .and. y?=w391:bool)
    n307 = And(x=w337, y=w336) -> (x .and. y?=w334:bool)
    n308 = Subtract(x=w329, y=w335) -> (x-y=w333:dbl)
    n309 = And(x=w350, y=w349) -> (x .and. y?=w347:bool)
    n310 = Subtract(x=w340, y=w348) -> (x-y=w346:dbl)
    n311 = And(x=w363, y=w362) -> (x .and. y?=w360:bool)
    n312 = Subtract(x=w343, y=w361) -> (x-y=w359:dbl)
    n313 = case shown="True" w384 {
      tunnel: w385 -> [_ w541]
      tunnel: [0.0 w541] -> w374
      frame False {
      }
      frame True {
      }
    }
    n314 = case shown="True" w413 {
      tunnel: w412 -> [_ w545]
      tunnel: [0.0 w545] -> w406
      frame False {
      }
      frame True {
      }
    }
    n315 = case shown="False" w439 {
      tunnel: w438 -> [_ w553]
      tunnel: [0.0 w553] -> w436
      frame False {
      }
      frame True {
      }
    }
    n316 = case shown="False" w428 {
      tunnel: w429 -> [_ w549]
      tunnel: [0.0 w549] -> w419
      frame False {
      }
      frame True {
      }
    }
    n317 = case shown="True" w402 {
      tunnel: w403 -> [_ w533]
      tunnel: [0.0 w533] -> w366
      frame False {
      }
      frame True {
      }
    }
    n318 = case shown="True" w141 {
      tunnel: w140 -> [_ w465]
      tunnel: [0.0 w465] -> w120
      frame False {
      }
      frame True {
      }
    }
    n319 = case shown="True" w391 {
      tunnel: w390 -> [_ w537]
      tunnel: [0.0 w537] -> w367
      frame False {
      }
      frame True {
      }
    }
    n320 = case shown="True" w155 {
      tunnel: w156 -> [_ w469]
      tunnel: [0.0 w469] -> w121
      frame False {
      }
      frame True {
      }
    }
    n321 = case shown="True" w131 {
      tunnel: w132 -> [_ w461]
      tunnel: [0.0 w461] -> w119
      frame False {
      }
      frame True {
      }
    }
    n322 = case shown="True" w239 {
      tunnel: w238 -> [_ w493]
      tunnel: [0.0 w493] -> w202
      frame False {
      }
      frame True {
      }
    }
    n323 = case shown="True" w217 {
      tunnel: w216 -> [_ w485]
      tunnel: [0.0 w485] -> w200
      frame False {
      }
      frame True {
      }
    }
    n324 = case shown="True" w231 {
      tunnel: w232 -> [_ w489]
      tunnel: [0.0 w489] -> w201
      frame False {
      }
      frame True {
      }
    }
    n325 = case shown="True" w256 {
      tunnel: w257 -> [_ w497]
      tunnel: [0.0 w497] -> w203
      frame False {
      }
      frame True {
      }
    }
    n326 = case shown="True" w296 {
      tunnel: w295 -> [_ w509]
      tunnel: [0.0 w509] -> w287
      frame False {
      }
      frame True {
      }
    }
    n327 = case shown="True" w265 {
      tunnel: w264 -> [_ w501]
      tunnel: [0.0 w501] -> w204
      frame False {
      }
      frame True {
      }
    }
    n328 = case shown="True" w308 {
      tunnel: w307 -> [_ w513]
      tunnel: [0.0 w513] -> w288
      frame False {
      }
      frame True {
      }
    }
    n329 = case shown="True" w183 {
      tunnel: w182 -> [_ w477]
      tunnel: [0.0 w477] -> w162
      frame False {
      }
      frame True {
      }
    }
    n330 = case shown="True" w280 {
      tunnel: w281 -> [_ w505]
      tunnel: [0.0 w505] -> w205
      frame False {
      }
      frame True {
      }
    }
    n331 = case shown="True" w320 {
      tunnel: w319 -> [_ w517]
      tunnel: [0.0 w517] -> w289
      frame False {
      }
      frame True {
      }
    }
    n332 = case shown="True" w334 {
      tunnel: w333 -> [_ w521]
      tunnel: [0.0 w521] -> w326
      frame False {
      }
      frame True {
      }
    }
    n333 = case shown="True" w194 {
      tunnel: w193 -> [_ w481]
      tunnel: [0.0 w481] -> w163
      frame False {
      }
      frame True {
      }
    }
    n334 = case shown="True" w347 {
      tunnel: w346 -> [_ w525]
      tunnel: [0.0 w525] -> w327
      frame False {
      }
      frame True {
      }
    }
    n335 = case shown="True" w170 {
      tunnel: w169 -> [_ w473]
      tunnel: [0.0 w473] -> w161
      frame False {
      }
      frame True {
      }
    }
    n336 = case shown="False" w360 {
      tunnel: w359 -> [_ w529]
      tunnel: [0.0 w529] -> w353
      frame False {
      }
      frame True {
      }
    }
    n337 = Build Array(w353, w327, w326, w289, w288, w287) -> (w354:dbl[])
    "7 Hz" <- w354
    n338 = Build Array(w436, w419, w406, w374, w367, w366) -> (w434:dbl[])
    "6 Hz" <- w434
    n339 = Array Max & Min(array=w354) -> (max value=w118:dbl, max index (indices)=→"Max Index 7":i32)  [unwired: 2 out]
    "PSD max 7" <- w118
    n340 = Array Max & Min(array=w434) -> (max value=w115:dbl, max index (indices)=→"Max Index 6":i32)  [unwired: 2 out]
    "PSD max 6" <- w115
    n341 = Build Array(w205, w204, w203, w202, w201, w200) -> (w206:dbl[])
    "8 Hz" <- w206
    n342 = Build Array(w163, w162, w161, w121, w120, w119) -> (w164:dbl[])
    "9 Hz" <- w164
    n343 = Array Max & Min(array=w206) -> (max value=w117:dbl, max index (indices)=→"Max Index 8":i32)  [unwired: 2 out]
    "PSD max 8" <- w117
    n344 = Array Max & Min(array=w164) -> (max value=w116:dbl, max index (indices)=→"Max Index 9":i32)  [unwired: 2 out]
    "PSD max 9" <- w116
    n345 = Build Array(w115, w118, w117, w116) -> (w114:dbl[])
    n346 = Array Max & Min(array=w114) -> (max value=w112:dbl, max index (indices)=w113:i32)  [unwired: 2 out]
    "max value" <- w112
    "PSD MAX" <- w112
    n347 = Greater?(x=w112, y=0.0 ("x")) -> (0:w110:bool)
    n348 = case shown="True" w110 {
      tunnel: w113 -> [_ w459]
      tunnel: [555 w459] -> w102
      frame False {
      }
      frame True {
      }
    }
    "Index ที่มากที่สุด" <- w102
    n349 = Equal?(x=0, y=w102) -> (x = y?=→"6 HZ 2" →"Emotion 4":bool)
    n350 = Equal?(x=1, y=w102) -> (x = y?=→"7 HZ" →"Emotion 5":bool)
    n351 = Equal?(x=2, y=w102) -> (x = y?=→"8 HZ" →"Emotion 6":bool)
    n352 = Equal?(x=3, y=w102) -> (x = y?=→"9 HZ" →"Emotion 7":bool)
    n353 = Equal?(x=555, y=w102) -> (x = y?=→"555":bool)
  }
  n354 = while {
    stop <- FALSE stop-if-true
    n355 = event shown="[4] \"Emer\": Value Change" {
      selector: _ -> [_ _ _ _ _ _ _]
      dyn-events: _ -> [_ _ _ _ _ _ _]
      timeout: _ -> [_ _ _ _ _ _ _]
      event Timeout {
        n356 = event-data() -> ()  [unwired: 1 in, 3 out]
      }
      event "commu": Value Change {
        n357 = event-data() -> ()  [unwired: 1 in, 6 out]
        n358 = local write "Tab Control"(enum32{"TAB 1", "TAB 2", "TAB 3", "TAB 4"}."TAB 2" ("Tab Control")) -> ()
      }
      event "call": Value Change {
        n359 = event-data() -> ()  [unwired: 1 in, 6 out]
        n360 = local write "Tab Control"(enum32{"TAB 1", "TAB 2", "TAB 3", "TAB 4"}."TAB 3" ("Tab Control")) -> ()
      }
      event "back_page2": Value Change {
        n361 = event-data() -> ()  [unwired: 1 in, 6 out]
        n362 = local write "Tab Control"(T3."TAB 1" ("Tab Control")) -> ()
      }
      event "Emer": Value Change {
        n363 = event-data() -> ()  [unwired: 1 in, 6 out]
        n364 = local write "Tab Control"(enum32{"TAB 1", "TAB 2", "TAB 3", "TAB 4"}."TAB 4" ("Tab Control")) -> ()
      }
      event "ele": Value Change {
        n365 = event-data() -> ()  [unwired: 1 in, 6 out]
        n366 = local write "Tab Control"(enum32{"TAB 1", "TAB 2", "TAB 3", "TAB 4"}."TAB 4" ("Tab Control")) -> ()
      }
      event "BACK_Page4": Value Change {
        n367 = event-data() -> ()  [unwired: 1 in, 6 out]
        n368 = local write "Tab Control"(enum32{"TAB 1", "TAB 2", "TAB 3", "TAB 4"}."TAB 1" ("Tab Control")) -> ()
      }
    }
  }
  n369 = local read "Tab Control"() -> (w2:enum32{"TAB 1", "TAB 2", "TAB 3", "TAB 4"})
  n370 = Obtain Notifier(notification data type=w2) -> (notifier out=w1:refnum<notifier>, error out=w4:errorcluster)  [unwired: 3 in, 1 out]
  n371 = while {
    tunnel: w1 -> [w573]
    stop <- FALSE stop-if-true
    n372 = Wait on Notification(notifier=w573) -> (notification=w572:enum32{"TAB 1", "TAB 2", "TAB 3", "TAB 4"})  [unwired: 3 in, 3 out]
    n373 = case shown="\"TAB 2\"" w572 {
      frame "TAB 1" {
        n374 = while {
          stop <- w594 stop-if-true
          n375 = flat-sequence {
            frame #0 {
              n376 = while {
                stop <- w597 stop-if-true
                n377 = local read "Clear1"() -> (w595:bool)
                n378 = local read "ele"() -> (w596:bool)
                n379 = Or(x=w596, y=w595) -> (x .or. y?=w597:bool)
              }
            }
            frame #1 {
              n380 = while {
                stop <- w603 stop-if-true
                n381 = local read "Index ที่มากที่สุด"() -> (w602:i32)
                n382 = Equal?(x=w602, y=0) -> (x = y?=→"ele":bool)
                n383 = local read "Clear1"() -> (w599:bool)
                n384 = local read "call"() -> (w600:bool)
                n385 = Or(x=w600, y=w599) -> (x .or. y?=w603:bool)
              }
            }
            frame #2 {
              n386 = while {
                stop <- w606 stop-if-true
                n387 = local read "Index ที่มากที่สุด"() -> (w609:i32)
                n388 = local read "commu"() -> (w604:bool)
                n389 = local read "Clear1"() -> (w605:bool)
                n390 = Equal?(x=w609, y=1) -> (x = y?=→"call":bool)
                n391 = Or(x=w604, y=w605) -> (x .or. y?=w606:bool)
              }
            }
            frame #3 {
              n392 = while {
                stop <- w610 stop-if-true
                n393 = local read "Index ที่มากที่สุด"() -> (w615:i32)
                n394 = local read "Clear1"() -> (w611:bool)
                n395 = local read "Emer"() -> (w612:bool)
                n396 = Equal?(x=w615, y=2) -> (x = y?=→"com":bool)
                n397 = Or(x=w612, y=w611) -> (x .or. y?=w610:bool)
              }
            }
          }
          n398 = local read "Clear1"() -> (w594:bool)
        }
        n399 = while {
          stop <- w625 stop-if-true
          n400 = local read "Baseline"() -> (w617:bool)
          n401 = case shown="True" w617 {
            tunnel: ["start" FALSE] -> w616
            frame False {
            }
            frame True {
            }
          }
          n402 = feedback #25() -> (w637:i32)  [unwired: 1 in]
          n403 = case shown="True" w616 {
            tunnel: [w663 w664] -> w638
            tunnel: w637 -> [w663 w665]
            frame False {
            }
            frame True {
              n404 = Increment(x=w665) -> (x+1=w664:i32)
            }
          }
          n405 = case shown="1" w638 {
            selector: w638 -> [w642 w646 w647 w654 w658 w661]
            tunnel: [w642 w646 w647 w654 w658 w660] -> w636
            frame 0, Default {
              w641 = FALSE ("B")
              n406 = local write "ele"(w641) -> ()
              n407 = local write "call"(w641) -> ()
              n408 = local write "commu"(w641) -> ()
              n409 = local write "Emotion"(w641) -> ()
              n410 = local write "Activity"(w641) -> ()
              n411 = local write "ACC"(w641) -> ()
            }
            frame 1 {
              n412 = local write "Emer"(FALSE) -> ()
              n413 = Wait (ms)(milliseconds to wait=u32 1500 ("millisecond timer value")) -> ()  [unwired: 1 out]
              "ele" <- TRUE
            }
            frame 2 {
              n414 = local write "ele"(FALSE) -> ()
              n415 = Wait (ms)(milliseconds to wait=u32 1000) -> ()  [unwired: 1 out]
              "call" <- TRUE
            }
            frame 3 {
              n416 = local write "call"(FALSE) -> ()
              n417 = Wait (ms)(milliseconds to wait=u32 1000) -> ()  [unwired: 1 out]
              "commu" <- TRUE
            }
            frame 4 {
              n418 = local write "commu"(FALSE) -> ()
              n419 = Wait (ms)(milliseconds to wait=u32 1000) -> ()  [unwired: 1 out]
              "Emer" <- TRUE
            }
            frame 5 {
              n420 = Subtract(x=w661, y=5 ("x")) -> (x-y=w660:i32)
              n421 = Wait (ms)(milliseconds to wait=u32 1200 ("millisecond timer value")) -> ()  [unwired: 1 out]
            }
          }
          n422 = feedback-in #25(w636) -> ()
          n423 = local read "Tab Control"() -> (w627:enum32{"TAB 1", "TAB 2", "TAB 3", "TAB 4"})
          n424 = Equal?(x=w627, y=T3."TAB 2" ("Tab Control")) -> (x = y?=w635:bool)
          n425 = Equal?(x=w627, y=T3."TAB 6" ("Tab Control")) -> (x = y?=w629:bool)
          n426 = Equal?(x=w627, y=T3."TAB 3" ("Tab Control")) -> (x = y?=w634:bool)
          n427 = Equal?(x=w627, y=T3."TAB 4" ("Tab Control")) -> (x = y?=w633:bool)
          n428 = Equal?(x=w627, y=T3."TAB 7" ("Tab Control")) -> (x = y?=w628:bool)
          n429 = Equal?(x=w627, y=T3."TAB 5" ("Tab Control")) -> (x = y?=w632:bool)
          n430 = Or(x=w635, y=w634) -> (x .or. y?=w631:bool)
          n431 = Or(x=w629, y=w628) -> (x .or. y?=w624:bool)
          n432 = Or(x=w633, y=w632) -> (x .or. y?=w630:bool)
          n433 = Or(x=w631, y=w630) -> (x .or. y?=w626:bool)
          n434 = Or(x=w626, y=w624) -> (x .or. y?=w625:bool)
        }
        n435 = while {
          stop <- w575 stop-if-true
          n436 = local read "Tab Control"() -> (w585:enum32{"TAB 1", "TAB 2", "TAB 3", "TAB 4"})
          n437 = Equal?(x=w585, y=T3."TAB 2" ("Tab Control")) -> (x = y?=w593:bool)
          n438 = Equal?(x=w585, y=T3."TAB 3" ("Tab Control")) -> (x = y?=w592:bool)
          n439 = Equal?(x=w585, y=T3."TAB 4" ("Tab Control")) -> (x = y?=w591:bool)
          n440 = Equal?(x=w585, y=T3."TAB 5" ("Tab Control")) -> (x = y?=w581:bool)
          n441 = Equal?(x=w585, y=T3."TAB 6" ("Tab Control")) -> (x = y?=w580:bool)
          n442 = Equal?(x=w585, y=T3."TAB 7" ("Tab Control")) -> (x = y?=w577:bool)
          n443 = Or(x=w593, y=w592) -> (x .or. y?=w590:bool)
          n444 = Or(x=w592, y=w591) -> (x .or. y?=w589:bool)
          n445 = Or(x=w581, y=w580) -> (x .or. y?=w578:bool)
          n446 = Or(x=w590, y=w589) -> (x .or. y?=w579:bool)
          n447 = Or(x=w578, y=w577) -> (x .or. y?=w576:bool)
          n448 = Or(x=w579, y=w576) -> (x .or. y?=w575:bool)
          "Clear1" <- w575
        }
      }
      frame "TAB 2" {
        n449 = while {
          stop <- w721 stop-if-true
          n450 = local read "start"() -> (w713:bool)
          n451 = feedback #26() -> (w733:i32)  [unwired: 1 in]
          n452 = case shown="True" w713 {
            tunnel: [w757 w758] -> w734
            tunnel: w733 -> [w757 w759]
            frame False {
            }
            frame True {
              n453 = Increment(x=w759) -> (x+1=w758:i32)
            }
          }
          n454 = case shown="2" w734 {
            selector: w734 -> [w736 w740 w743 w748 w752 w755]
            tunnel: [w736 w740 w743 w748 w752 w754] -> w732
            frame 0, Default {
              w735 = FALSE ("B")
              n455 = local write "commu_back"(w735) -> ()
              n456 = local write "commu_2"(w735) -> ()
              n457 = local write "commu_1"(w735) -> ()
              n458 = local write "8-2"(w735) -> ()
            }
            frame 1 {
              n459 = local write "commu_back"(FALSE) -> ()
              n460 = Wait (ms)(milliseconds to wait=u32 1500 ("millisecond timer value")) -> ()  [unwired: 1 out]
              "commu_1" <- TRUE
            }
            frame 2 {
              n461 = local write "commu_1"(FALSE) -> ()
              n462 = Wait (ms)(milliseconds to wait=u32 1000) -> ()  [unwired: 1 out]
              "commu_2" <- TRUE
            }
            frame 3 {
              n463 = local write "commu_2"(FALSE) -> ()
              n464 = Wait (ms)(milliseconds to wait=u32 1000) -> ()  [unwired: 1 out]
              "8-2" <- TRUE
            }
            frame 4 {
              n465 = local write "8-2"(FALSE) -> ()
              n466 = Wait (ms)(milliseconds to wait=u32 1000) -> ()  [unwired: 1 out]
              "commu_back" <- TRUE
            }
            frame 5 {
              n467 = Subtract(x=w755, y=5 ("x")) -> (x-y=w754:i32)
              n468 = Wait (ms)(milliseconds to wait=u32 1200 ("millisecond timer value")) -> ()  [unwired: 1 out]
            }
          }
          n469 = feedback-in #26(w732) -> ()
          n470 = local read "Tab Control"() -> (w723:enum32{"TAB 1", "TAB 2", "TAB 3", "TAB 4"})
          n471 = Equal?(x=w723, y=T3."TAB 1" ("Tab Control")) -> (x = y?=w731:bool)
          n472 = Equal?(x=w723, y=T3."TAB 6" ("Tab Control")) -> (x = y?=w725:bool)
          n473 = Equal?(x=w723, y=T3."TAB 3" ("Tab Control")) -> (x = y?=w730:bool)
          n474 = Equal?(x=w723, y=T3."TAB 4" ("Tab Control")) -> (x = y?=w729:bool)
          n475 = Equal?(x=w723, y=T3."TAB 7" ("Tab Control")) -> (x = y?=w724:bool)
          n476 = Equal?(x=w723, y=T3."TAB 5" ("Tab Control")) -> (x = y?=w728:bool)
          n477 = Or(x=w731, y=w730) -> (x .or. y?=w727:bool)
          n478 = Or(x=w725, y=w724) -> (x .or. y?=w720:bool)
          n479 = Or(x=w729, y=w728) -> (x .or. y?=w726:bool)
          n480 = Or(x=w727, y=w726) -> (x .or. y?=w722:bool)
          n481 = Or(x=w722, y=w720) -> (x .or. y?=w721:bool)
        }
        n482 = while {
          stop <- w685 stop-if-true
          n483 = flat-sequence {
            frame #0 {
              n484 = while {
                stop <- w688 stop-if-true
                n485 = local read "commu_1"() -> (w686:bool)
                n486 = local read "Clear2"() -> (w687:bool)
                n487 = Or(x=w686, y=w687) -> (x .or. y?=w688:bool)
              }
            }
            frame #1 {
              n488 = while {
                stop <- w694 stop-if-true
                n489 = local read "Index ที่มากที่สุด"() -> (w693:i32)
                n490 = local read "commu_2"() -> (w689:bool)
                n491 = local read "Clear2"() -> (w691:bool)
                n492 = Equal?(x=w693, y=0) -> (x = y?=→"Activity":bool)
                n493 = Or(x=w689, y=w691) -> (x .or. y?=w694:bool)
              }
            }
            frame #2 {
              n494 = while {
                stop <- w698 stop-if-true
                n495 = local read "Index ที่มากที่สุด"() -> (w700:i32)
                n496 = local read "Clear2"() -> (w697:bool)
                n497 = local read "8-2"() -> (w695:bool)
                n498 = Equal?(x=w700, y=1) -> (x = y?=→"Emotion":bool)
                n499 = Or(x=w695, y=w697) -> (x .or. y?=w698:bool)
              }
            }
            frame #3 {
              n500 = while {
                stop <- w703 stop-if-true
                n501 = local read "Index ที่มากที่สุด"() -> (w706:i32)
                n502 = local read "commu_back"() -> (w701:bool)
                n503 = local read "Clear2"() -> (w704:bool)
                n504 = Equal?(x=w706, y=2) -> (x = y?=→"ACC":bool)
                n505 = Or(x=w701, y=w704) -> (x .or. y?=w703:bool)
              }
            }
            frame #4 {
              n506 = while {
                stop <- FALSE stop-if-true
                n507 = local read "Index ที่มากที่สุด"() -> (w712:i32)
                n508 = local read "commu_1"() -> (w708:bool)
                n509 = local read "Clear2"() -> (w709:bool)
                n510 = Equal?(x=w712, y=3) -> (x = y?=→"back_page2":bool)
                n511 = Or(x=w708, y=w709) -> ()  [unwired: 1 out]
              }
            }
          }
          n512 = local read "Clear2"() -> (w685:bool)
        }
        n513 = while {
          stop <- w666 stop-if-true
          n514 = local read "Tab Control"() -> (w676:enum32{"TAB 1", "TAB 2", "TAB 3", "TAB 4"})
          n515 = Equal?(x=w676, y=T3."TAB 1" ("Tab Control")) -> (x = y?=w684:bool)
          n516 = Equal?(x=w676, y=T3."TAB 3" ("Tab Control")) -> (x = y?=w683:bool)
          n517 = Equal?(x=w676, y=T3."TAB 4" ("Tab Control")) -> (x = y?=w682:bool)
          n518 = Equal?(x=w676, y=T3."TAB 5" ("Tab Control")) -> (x = y?=w672:bool)
          n519 = Equal?(x=w676, y=T3."TAB 6" ("Tab Control")) -> (x = y?=w671:bool)
          n520 = Equal?(x=w676, y=T3."TAB 7" ("Tab Control")) -> (x = y?=w668:bool)
          n521 = Or(x=w684, y=w683) -> (x .or. y?=w681:bool)
          n522 = Or(x=w683, y=w682) -> (x .or. y?=w680:bool)
          n523 = Or(x=w672, y=w671) -> (x .or. y?=w669:bool)
          n524 = Or(x=w681, y=w680) -> (x .or. y?=w670:bool)
          n525 = Or(x=w669, y=w668) -> (x .or. y?=w667:bool)
          n526 = Or(x=w670, y=w667) -> (x .or. y?=w666:bool)
          "Clear2" <- w666
        }
        n527 = call "Elapsed Time"() -> ()  [unwired: 12 in, 8 out]
      }
      frame "TAB 3" {
        n528 = while {
          stop <- w815 stop-if-true
          n529 = local read "start"() -> (w807:bool)
          n530 = feedback #27() -> (w827:i32)  [unwired: 1 in]
          n531 = case shown="True" w807 {
            tunnel: [w851 w852] -> w828
            tunnel: w827 -> [w851 w853]
            frame False {
            }
            frame True {
              n532 = Increment(x=w853) -> (x+1=w852:i32)
            }
          }
          n533 = case shown="1" w828 {
            selector: w828 -> [w830 w834 w837 w842 w846 w849]
            tunnel: [w830 w834 w837 w842 w846 w848] -> w826
            frame 0, Default {
              w829 = FALSE ("B")
              n534 = local write "call_back"(w829) -> ()
              n535 = local write "call_1"(w829) -> ()
              n536 = local write "call_2"(w829) -> ()
              n537 = local write "call_3"(w829) -> ()
            }
            frame 1 {
              n538 = local write "call_back"(FALSE) -> ()
              n539 = Wait (ms)(milliseconds to wait=u32 1500 ("millisecond timer value")) -> ()  [unwired: 1 out]
              "call_1" <- TRUE
            }
            frame 2 {
              n540 = local write "call_1"(FALSE) -> ()
              n541 = Wait (ms)(milliseconds to wait=u32 1000) -> ()  [unwired: 1 out]
              "call_2" <- TRUE
            }
            frame 3 {
              n542 = local write "call_2"(FALSE) -> ()
              n543 = Wait (ms)(milliseconds to wait=u32 1000) -> ()  [unwired: 1 out]
              "call_3" <- TRUE
            }
            frame 4 {
              n544 = local write "call_3"(FALSE) -> ()
              n545 = Wait (ms)(milliseconds to wait=u32 1000) -> ()  [unwired: 1 out]
              "call_back" <- TRUE
            }
            frame 5 {
              n546 = Subtract(x=w849, y=5 ("x")) -> (x-y=w848:i32)
              n547 = Wait (ms)(milliseconds to wait=u32 1200 ("millisecond timer value")) -> ()  [unwired: 1 out]
            }
          }
          n548 = feedback-in #27(w826) -> ()
          n549 = local read "Tab Control"() -> (w817:enum32{"TAB 1", "TAB 2", "TAB 3", "TAB 4"})
          n550 = Equal?(x=w817, y=T3."TAB 1" ("Tab Control")) -> (x = y?=w825:bool)
          n551 = Equal?(x=w817, y=T3."TAB 6" ("Tab Control")) -> (x = y?=w819:bool)
          n552 = Equal?(x=w817, y=T3."TAB 2" ("Tab Control")) -> (x = y?=w824:bool)
          n553 = Equal?(x=w817, y=T3."TAB 4" ("Tab Control")) -> (x = y?=w823:bool)
          n554 = Equal?(x=w817, y=T3."TAB 7" ("Tab Control")) -> (x = y?=w818:bool)
          n555 = Equal?(x=w817, y=T3."TAB 5" ("Tab Control")) -> (x = y?=w822:bool)
          n556 = Or(x=w825, y=w824) -> (x .or. y?=w821:bool)
          n557 = Or(x=w819, y=w818) -> (x .or. y?=w814:bool)
          n558 = Or(x=w823, y=w822) -> (x .or. y?=w820:bool)
          n559 = Or(x=w821, y=w820) -> (x .or. y?=w816:bool)
          n560 = Or(x=w816, y=w814) -> (x .or. y?=w815:bool)
        }
        n561 = while {
          stop <- w779 stop-if-true
          n562 = flat-sequence {
            frame #0 {
              n563 = while {
                stop <- w782 stop-if-true
                n564 = local read "Clear 3"() -> (w781:bool)
                n565 = local read "call_1"() -> (w780:bool)
                n566 = Or(x=w780, y=w781) -> (x .or. y?=w782:bool)
              }
            }
            frame #1 {
              n567 = while {
                stop <- w788 stop-if-true
                n568 = local read "Index ที่มากที่สุด"() -> (w787:i32)
                n569 = local read "Clear 3"() -> (w783:bool)
                n570 = local read "call_2"() -> (w784:bool)
                n571 = Equal?(x=w787, y=0) -> (x = y?=→"1":bool)
                n572 = Or(x=w784, y=w783) -> (x .or. y?=w788:bool)
              }
            }
            frame #2 {
              n573 = while {
                stop <- w789 stop-if-true
                n574 = local read "Index ที่มากที่สุด"() -> (w794:i32)
                n575 = local read "Clear 3"() -> (w791:bool)
                n576 = local read "call_3"() -> (w790:bool)
                n577 = Equal?(x=w794, y=1) -> (x = y?=→"1 2":bool)
                n578 = Or(x=w790, y=w791) -> (x .or. y?=w789:bool)
              }
            }
            frame #3 {
              n579 = while {
                stop <- w798 stop-if-true
                n580 = local read "Index ที่มากที่สุด"() -> (w800:i32)
                n581 = local read "call_back"() -> (w795:bool)
                n582 = local read "Clear 3"() -> (w796:bool)
                n583 = Equal?(x=w800, y=2) -> (x = y?=→"1 3":bool)
                n584 = Or(x=w795, y=w796) -> (x .or. y?=w798:bool)
              }
            }
            frame #4 {
              n585 = while {
                stop <- FALSE stop-if-true
                n586 = local read "Index ที่มากที่สุด"() -> (w806:i32)
                n587 = local read "call_1"() -> (w801:bool)
                n588 = local read "Clear 3"() -> (w802:bool)
                n589 = Equal?(x=w806, y=3) -> (x = y?=→"call_back":bool)
                n590 = Or(x=w801, y=w802) -> ()  [unwired: 1 out]
              }
            }
          }
          n591 = local read "Clear 3"() -> (w779:bool)
        }
        n592 = while {
          stop <- w760 stop-if-true
          n593 = local read "Tab Control"() -> (w770:enum32{"TAB 1", "TAB 2", "TAB 3", "TAB 4"})
          n594 = Equal?(x=w770, y=T3."TAB 1" ("Tab Control")) -> (x = y?=w778:bool)
          n595 = Equal?(x=w770, y=T3."TAB 2" ("Tab Control")) -> (x = y?=w777:bool)
          n596 = Equal?(x=w770, y=T3."TAB 4" ("Tab Control")) -> (x = y?=w776:bool)
          n597 = Equal?(x=w770, y=T3."TAB 5" ("Tab Control")) -> (x = y?=w766:bool)
          n598 = Equal?(x=w770, y=T3."TAB 6" ("Tab Control")) -> (x = y?=w765:bool)
          n599 = Equal?(x=w770, y=T3."TAB 7" ("Tab Control")) -> (x = y?=w762:bool)
          n600 = Or(x=w778, y=w777) -> (x .or. y?=w775:bool)
          n601 = Or(x=w777, y=w776) -> (x .or. y?=w774:bool)
          n602 = Or(x=w766, y=w765) -> (x .or. y?=w763:bool)
          n603 = Or(x=w775, y=w774) -> (x .or. y?=w764:bool)
          n604 = Or(x=w763, y=w762) -> (x .or. y?=w761:bool)
          n605 = Or(x=w764, y=w761) -> (x .or. y?=w760:bool)
          "Clear 3" <- w760
        }
      }
      frame "TAB 4" {
        n606 = while {
          stop <- w909 stop-if-true
          n607 = local read "start"() -> (w901:bool)
          n608 = feedback #28() -> (w921:i32)  [unwired: 1 in]
          n609 = case shown="True" w901 {
            tunnel: [w945 w946] -> w922
            tunnel: w921 -> [w945 w947]
            frame False {
            }
            frame True {
              n610 = Increment(x=w947) -> (x+1=w946:i32)
            }
          }
          n611 = case shown="1" w922 {
            selector: w922 -> [w924 w928 w931 w936 w940 w943]
            tunnel: [w924 w928 w931 w936 w940 w942] -> w920
            frame 0, Default {
              w923 = FALSE ("B")
              n612 = local write "ele_back"(w923) -> ()
              n613 = local write "ele_1"(w923) -> ()
              n614 = local write "ele_2"(w923) -> ()
              n615 = local write "ele_3"(w923) -> ()
            }
            frame 1 {
              n616 = local write "ele_back"(FALSE) -> ()
              n617 = Wait (ms)(milliseconds to wait=u32 1500 ("millisecond timer value")) -> ()  [unwired: 1 out]
              "ele_1" <- TRUE
            }
            frame 2 {
              n618 = local write "ele_1"(FALSE) -> ()
              n619 = Wait (ms)(milliseconds to wait=u32 1000) -> ()  [unwired: 1 out]
              "ele_2" <- TRUE
            }
            frame 3 {
              n620 = local write "ele_2"(FALSE) -> ()
              n621 = Wait (ms)(milliseconds to wait=u32 1000) -> ()  [unwired: 1 out]
              "ele_3" <- TRUE
            }
            frame 4 {
              n622 = local write "ele_3"(FALSE) -> ()
              n623 = Wait (ms)(milliseconds to wait=u32 1000) -> ()  [unwired: 1 out]
              "ele_back" <- TRUE
            }
            frame 5 {
              n624 = Subtract(x=w943, y=5 ("x")) -> (x-y=w942:i32)
              n625 = Wait (ms)(milliseconds to wait=u32 1200 ("millisecond timer value")) -> ()  [unwired: 1 out]
            }
          }
          n626 = feedback-in #28(w920) -> ()
          n627 = local read "Tab Control"() -> (w911:enum32{"TAB 1", "TAB 2", "TAB 3", "TAB 4"})
          n628 = Equal?(x=w911, y=T3."TAB 1" ("Tab Control")) -> (x = y?=w919:bool)
          n629 = Equal?(x=w911, y=T3."TAB 6" ("Tab Control")) -> (x = y?=w913:bool)
          n630 = Equal?(x=w911, y=T3."TAB 2" ("Tab Control")) -> (x = y?=w918:bool)
          n631 = Equal?(x=w911, y=T3."TAB 3" ("Tab Control")) -> (x = y?=w917:bool)
          n632 = Equal?(x=w911, y=T3."TAB 7" ("Tab Control")) -> (x = y?=w912:bool)
          n633 = Equal?(x=w911, y=T3."TAB 5" ("Tab Control")) -> (x = y?=w916:bool)
          n634 = Or(x=w919, y=w918) -> (x .or. y?=w915:bool)
          n635 = Or(x=w913, y=w912) -> (x .or. y?=w908:bool)
          n636 = Or(x=w917, y=w916) -> (x .or. y?=w914:bool)
          n637 = Or(x=w915, y=w914) -> (x .or. y?=w910:bool)
          n638 = Or(x=w910, y=w908) -> (x .or. y?=w909:bool)
        }
        n639 = while {
          stop <- w873 stop-if-true
          n640 = flat-sequence {
            frame #0 {
              n641 = while {
                stop <- w876 stop-if-true
                n642 = local read "Clear4"() -> (w875:bool)
                n643 = local read "ele_1"() -> (w874:bool)
                n644 = Or(x=w874, y=w875) -> (x .or. y?=w876:bool)
              }
            }
            frame #1 {
              n645 = while {
                stop <- w882 stop-if-true
                n646 = local read "Index ที่มากที่สุด"() -> (w881:i32)
                n647 = local read "Clear4"() -> (w879:bool)
                n648 = local read "ele_2"() -> (w877:bool)
                n649 = Equal?(x=w881, y=0) -> (x = y?=→"ele_1":bool)
                n650 = Or(x=w877, y=w879) -> (x .or. y?=w882:bool)
              }
            }
            frame #2 {
              n651 = while {
                stop <- w885 stop-if-true
                n652 = local read "Index ที่มากที่สุด"() -> (w888:i32)
                n653 = local read "Clear4"() -> (w886:bool)
                n654 = local read "ele_3"() -> (w883:bool)
                n655 = Equal?(x=w888, y=1) -> (x = y?=→"ele_2":bool)
                n656 = Or(x=w883, y=w886) -> (x .or. y?=w885:bool)
              }
            }
            frame #3 {
              n657 = while {
                stop <- w892 stop-if-true
                n658 = local read "Index ที่มากที่สุด"() -> (w894:i32)
                n659 = local read "ele_back"() -> (w889:bool)
                n660 = local read "Clear4"() -> (w891:bool)
                n661 = Equal?(x=w894, y=2) -> (x = y?=→"ele_3":bool)
                n662 = Or(x=w889, y=w891) -> (x .or. y?=w892:bool)
              }
            }
            frame #4 {
              n663 = while {
                stop <- FALSE stop-if-true
                n664 = local read "Index ที่มากที่สุด"() -> (w900:i32)
                n665 = local read "Clear4"() -> (w897:bool)
                n666 = local read "ele_1"() -> (w895:bool)
                n667 = Equal?(x=w900, y=3) -> (x = y?=→"BACK_Page4":bool)
                n668 = Or(x=w895, y=w897) -> ()  [unwired: 1 out]
              }
            }
          }
          n669 = local read "Clear4"() -> (w873:bool)
        }
        n670 = while {
          stop <- w854 stop-if-true
          n671 = local read "Tab Control"() -> (w864:enum32{"TAB 1", "TAB 2", "TAB 3", "TAB 4"})
          n672 = Equal?(x=w864, y=T3."TAB 1" ("Tab Control")) -> (x = y?=w872:bool)
          n673 = Equal?(x=w864, y=T3."TAB 2" ("Tab Control")) -> (x = y?=w871:bool)
          n674 = Equal?(x=w864, y=T3."TAB 3" ("Tab Control")) -> (x = y?=w870:bool)
          n675 = Equal?(x=w864, y=T3."TAB 5" ("Tab Control")) -> (x = y?=w860:bool)
          n676 = Equal?(x=w864, y=T3."TAB 6" ("Tab Control")) -> (x = y?=w859:bool)
          n677 = Equal?(x=w864, y=T3."TAB 7" ("Tab Control")) -> (x = y?=w856:bool)
          n678 = Or(x=w872, y=w871) -> (x .or. y?=w869:bool)
          n679 = Or(x=w871, y=w870) -> (x .or. y?=w868:bool)
          n680 = Or(x=w860, y=w859) -> (x .or. y?=w857:bool)
          n681 = Or(x=w869, y=w868) -> (x .or. y?=w858:bool)
          n682 = Or(x=w857, y=w856) -> (x .or. y?=w855:bool)
          n683 = Or(x=w858, y=w855) -> (x .or. y?=w854:bool)
          "Clear4" <- w854
        }
      }
    }
  }
  n684 = while {
    tunnel: w1 -> [w952]
    tunnel: [w951] -> w5
    tunnel: w4 -> [w950]
    tunnel: [w949] -> w3
    stop <- FALSE stop-if-true
    n685 = case shown="\"TAB 1\", Default" "Tab Control" {
      selector: "Tab Control" -> [w956 w980 w989 w998]
      tunnel: [w955 w977 w986 w996] -> w948
      frame "TAB 1", Default {
        n686 = local read "Index ที่มากที่สุด"() -> (w957:i32)
        n687 = local read "commu"() -> (w958:bool)
        n688 = Add(x=w956, y=3) -> (x+y=w975:u32)
        n689 = local read "Index ที่มากที่สุด"() -> (w963:i32)
        n690 = local read "Index ที่มากที่สุด"() -> (w961:i32)
        n691 = local read "ele"() -> (w962:bool)
        n692 = Equal?(x=w957, y=2) -> (x = y?=w973:bool)
        n693 = Increment(x=w956) -> (x+1=w967:enum32{"TAB 1", "TAB 2", "TAB 3", "TAB 4"})
        n694 = local read "call"() -> (w960:bool)
        n695 = And(x=w958, y=w973) -> (x .and. y?=w974:bool)
        n696 = Equal?(x=w963, y=0) -> (x = y?=w971:bool)
        n697 = Equal?(x=w961, y=1) -> (x = y?=w972:bool)
        n698 = And(x=w960, y=w972) -> (x .and. y?=w968:bool)
        n699 = And(x=w962, y=w971) -> (x .and. y?=w969:bool)
        n700 = Select(t=w975, s=w974, f=w956) -> (s? t:f=w976:u32)
        n701 = Select(t=w975, s=w968, f=w976) -> (s? t:f=w970:u32)
        n702 = Select(t=w967, s=w969, f=w970) -> (s? t:f=w955:u32)
      }
      frame "TAB 2" {
        n703 = local read "Index ที่มากที่สุด"() -> (w983:i32)
        n704 = local read "back_page2"() -> (w984:bool)
        n705 = Decrement(x=w980) -> (x-1=w982:enum32{"TAB 1", "TAB 2", "TAB 3", "TAB 4"})
        n706 = Equal?(x=w983, y=3) -> (x = y?=w979:bool)
        n707 = Not(x=w979) -> (.not. x?=w978:bool)
        n708 = And(x=w984, y=w979) -> (x .and. y?=w981:bool)
        n709 = local write "commu"(w978) -> ()
        n710 = Select(t=w982, s=w981, f=w980) -> (s? t:f=w977:enum32{"TAB 1", "TAB 2", "TAB 3", "TAB 4"})
      }
      frame "TAB 3" {
        n711 = local read "Index ที่มากที่สุด"() -> (w994:i32)
        n712 = local read "call_back"() -> (w991:bool)
        n713 = Subtract(x=w989, y=2) -> (x-y=w987:u32)
        n714 = Equal?(x=w994, y=3) -> (x = y?=w992:bool)
        n715 = And(x=w991, y=w992) -> (x .and. y?=w993:bool)
        n716 = Not(x=w992) -> (.not. x?=w990:bool)
        n717 = local write "call"(w990) -> ()
        n718 = Select(t=w987, s=w993, f=w989) -> (s? t:f=w986:u32)
      }
      frame "TAB 4" {
        n719 = local read "Index ที่มากที่สุด"() -> (w1004:i32)
        n720 = local read "BACK_Page4"() -> (w1001:bool)
        n721 = Subtract(x=w998, y=3) -> (x-y=w997:u32)
        n722 = Equal?(x=w1004, y=3) -> (x = y?=w1002:bool)
        n723 = And(x=w1001, y=w1002) -> (x .and. y?=w1003:bool)
        n724 = Not(x=w1002) -> (.not. x?=w1000:bool)
        n725 = local write "ele"(w1000) -> ()
        n726 = Select(t=w997, s=w1003, f=w998) -> (s? t:f=w996:u32)
      }
    }
    n727 = local write "Tab Control"(w948) -> ()
    n728 = Send Notification(notification=w948, notifier=w952, error in (no error)=w950) -> (notifier out=w951:refnum<notifier>, error out=w949:errorcluster)
  }
  n729 = Release Notifier(notifier=w5, error in (no error)=w3) -> ()  [unwired: 1 in, 3 out]
  n730 = call <vilib>:"Draw Flattened Pixmap.vi"() -> ()  [unwired: 9 in, 1 out]
  n731 = call <vilib>:"Draw Flattened Pixmap.vi"() -> ()  [unwired: 9 in, 1 out]
  n732 = call <vilib>:"Draw Flattened Pixmap.vi"() -> ()  [unwired: 9 in, 1 out]
